vi "Main.vi"() -> ()   [LabVIEW 2020]
uses:
  <vilib>/MakerHub/PS4-Controller/Private/Type Defs/Buttons.ctl
  <vilib>/MakerHub/PS4-Controller/Private/Type Defs/Axis.ctl
  <vilib>/MakerHub/PS4-Controller/Private/Type Defs/Indicators/DPad Enum.ctl
  C:/Users/Public/Documents/Photometrics/PMQI-LabViewSamples/Examples/2018/Dependencies/PVCamNET.dll
  Public/Documents/Photometrics/PMQI-LabViewSamples/Examples/2018/Dependencies/PVCamNET.dll
  <vilib>/SmarAct/SmarActCTL/SA_CTL.lvclass
  <vilib>/MakerHub/PS4-Controller/Private/Type Defs/PS4 Controller Ref.ctl
  <vilib>/Platform/TimedLoop/XDataNode/timing_clust.ctl
  <vilib>/Platform/TimedLoop/XDataNode/nitl_modes.ctl
  <vilib>/Platform/TimedLoop/XDataNode/wakeup.ctl
  <vilib>/platform/TimedLoop/XDataNode/XDataNode.xnode
  <vilib>/Platform/TimedLoop/XDataNode/XDNodeRunTimeDep.lvlib
  <vilib>/MakerHub/PS4-Controller/LMH-PS4.lvlib
panel:
  out "indicator_move_index":dbl
  out "indicator_error":i16
  out "error out 2":errorcluster
  out "indicator_control_sequence":bool=TRUE
  out "indicator_detector_intensity":string="0"
  out "indicator_acquisition_start_time":dbl
  out "indicator_UV_activation_time":dbl
  out "indicator_UV_activation_intensity":dbl
  out "time_out_of_focus":u64 caption="Phidget ID"
  out "indicator_focus_cycle":dbl
  out "indicator_positioner_current_position":i64[](array[numeric])
  out "indicator_focus_searching":bool=TRUE
  out "indicator_focus_userlocked":bool=TRUE
  out "indicator_image_width":u64 caption="Phidget ID"
  out "indicator_LED_power":u64 caption="Phidget ID"
  out "indicator_initial_position_y":u64 caption="Phidget ID"
  out "indicator_initial_position_x":u64 caption="Phidget ID"
  out "indicator_folder_path":string
  out "indicator_saved_positions":i64[][](array[numeric])
  out "indicator_current_position_index":u64 caption="Phidget ID"
  out "indicator_light_source_power":string="2.0"
  out "indicator_red_laser_power":u64 caption="Phidget ID"
  out "indicator_green_laser_power":u64 caption="Phidget ID"
  out "indicator_blue_laser_power":u64 caption="Phidget ID"
  out "indicator_violet_laser_power":u64 caption="Phidget ID"
  out "indicator_current_folder":u64 caption="Phidget ID"
  out "indicator_sequence_distance_y":dbl
  out "indicator_sequence_distance_x":dbl
  out "indicator_sequence_move_y":bool
  out "indicator_sequence_move_x":bool
  out "indicator_current_filter_index":u64 caption="Phidget ID"
  out "indicator_main_positioner_moving_x_y":bool
  in  "control_light_source":string
  out "indicator_devices_reference":T2
  out "indicator_sequence_current_parameters":T3
  out "indicator_sequence_parameters":T4
  out "indicator_camera_buffer_index":u64 caption="Phidget ID"
  in  "control_detector_serial_number":string="69251713"
  out "indicator_joystick_axes":T5
  out "indicator_joystick_buttons":T7
  in  "Stop":bool=TRUE
  out "indicator_main_all_devices_connected":bool
  out "indicator_main_detector_status":bool
  out "indicator_main_filter_status":bool
  out "indicator_main_joystick_status":bool
  out "indicator_main_light sources_status":bool
  out "indicator_main_positioner_status":bool
  out "indicator_main_camera_status":bool
  in  "control_saving_path":path
  out "indicator_message":string="Ready"
  in  "control_frames":string="1000"
  in  "control_sequence":bool
  in  "control_sequence_file_path":path
  in  "control_exposure":string="50"
  out "indicator_focus_status":string="Unfocused"
  out "indicator_x":string
  out "indicator_y":string
  out "indicator_z":string
  out "indicator_light_source":string="Red"
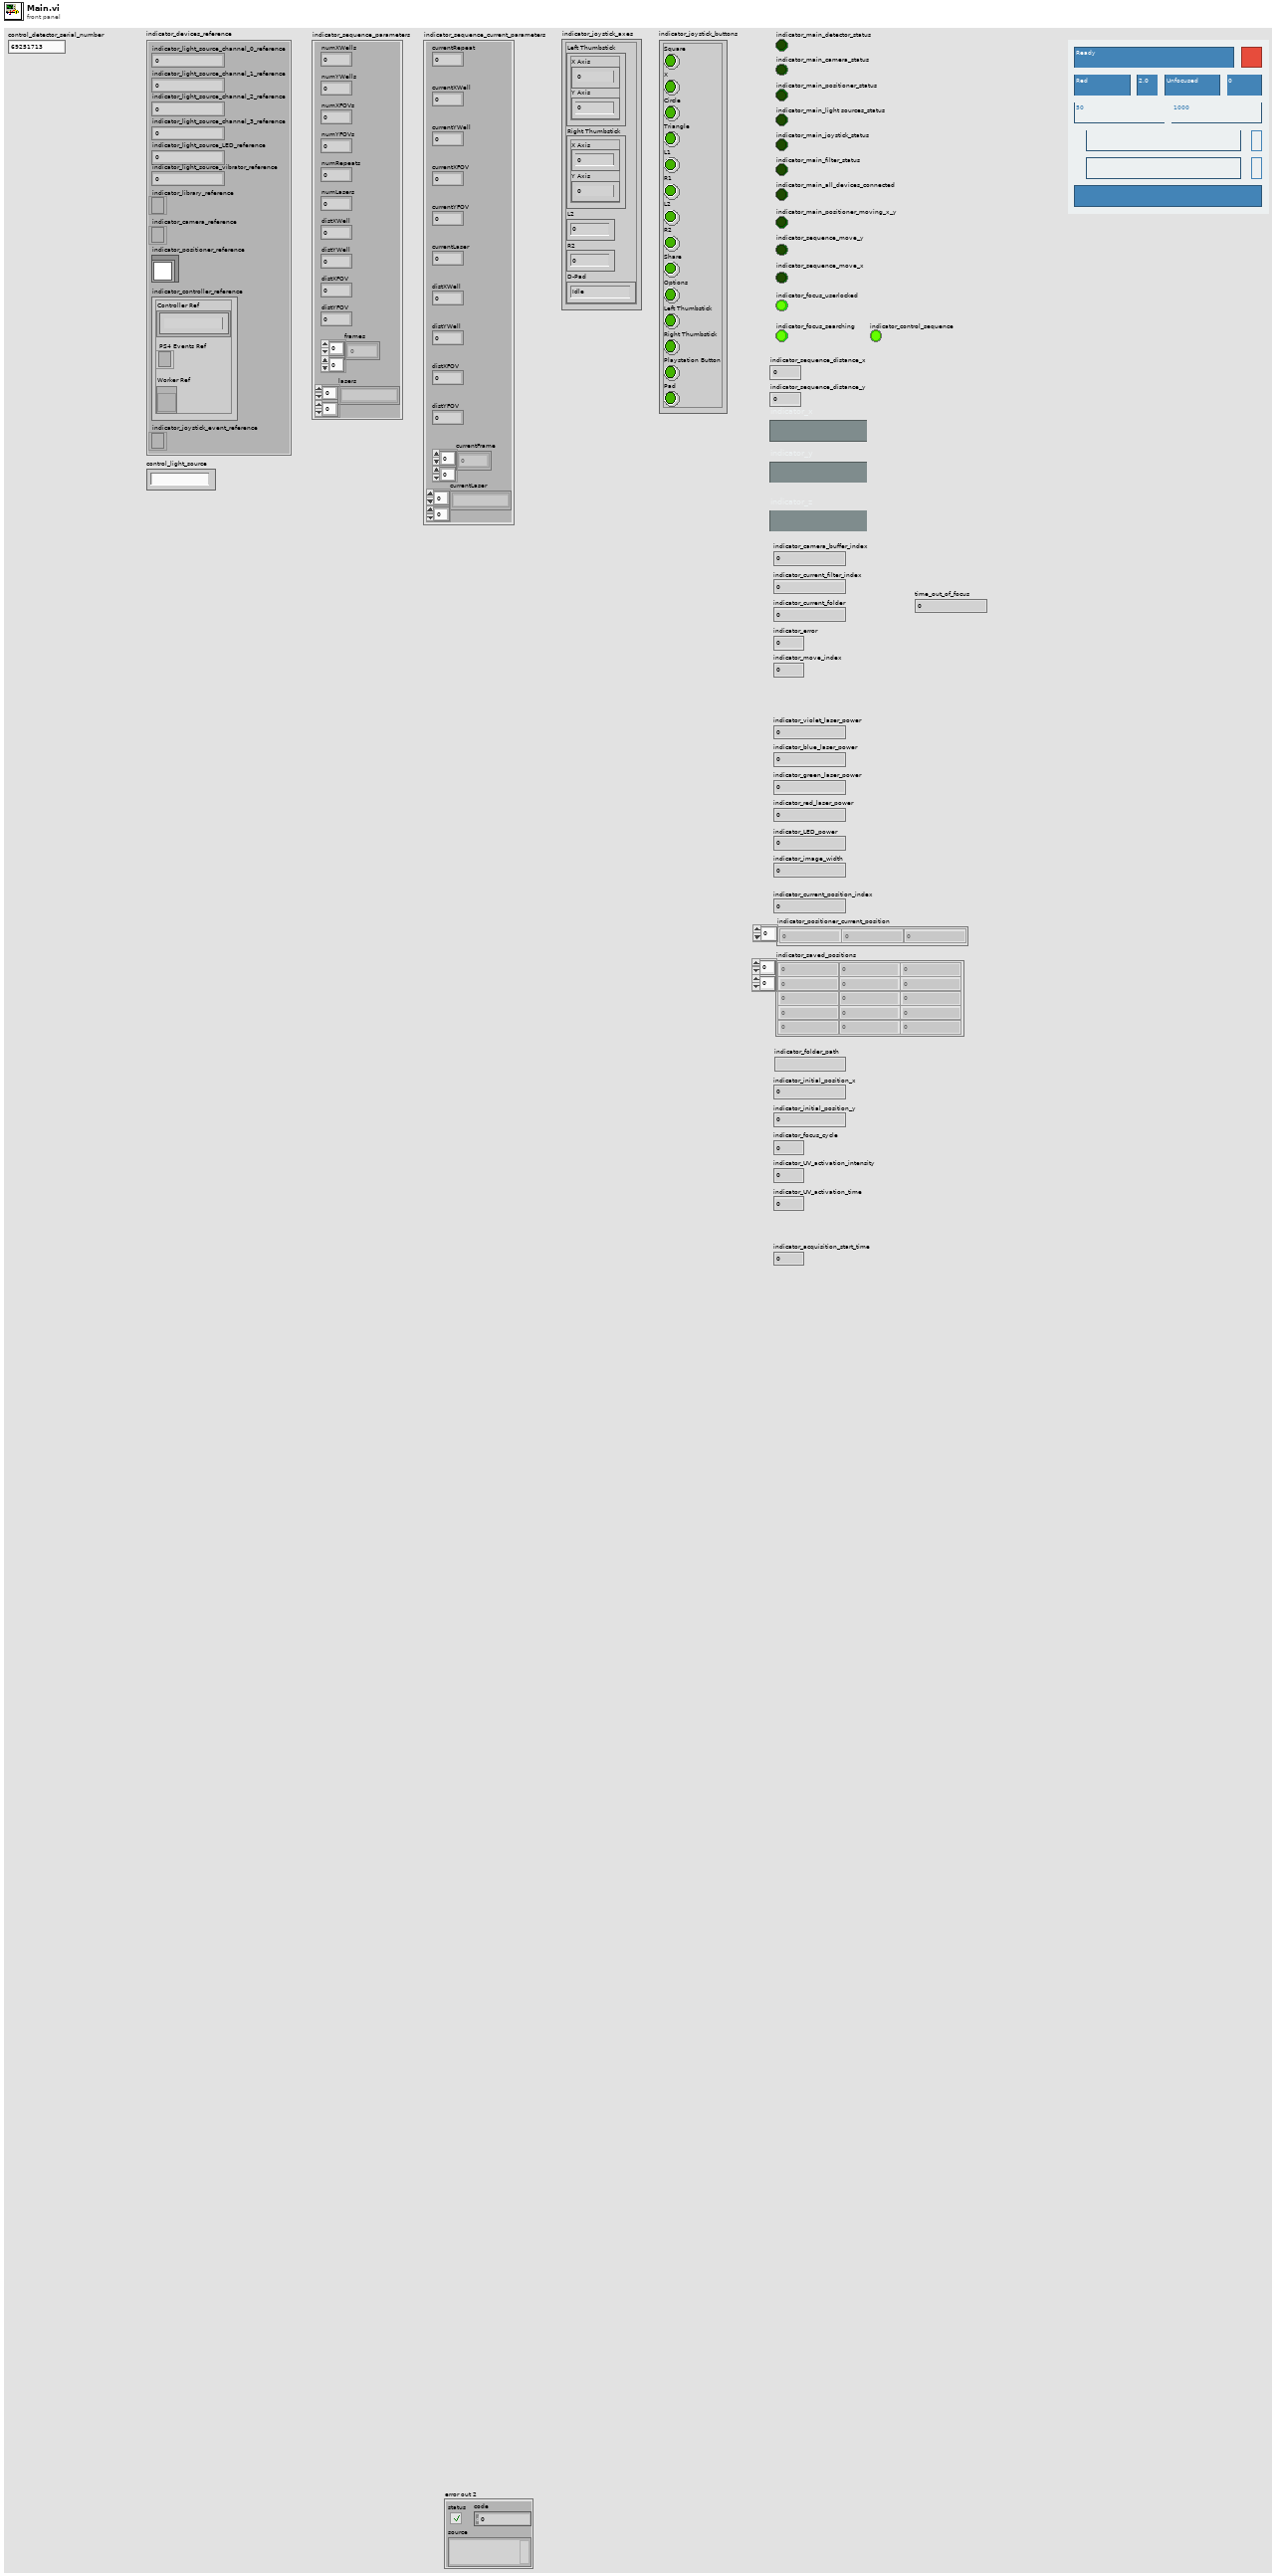
[diagram p1: front panel]
types:
  T1 = typedef "LMH-PS4.lvlib/PS4 Controller Ref.ctl" = cluster{"Controller Ref":refnum<k1>, "PS4 Events Ref":refnum<event-registration>, "Worker Ref":refnum<vi>}
  T2 = cluster{"indicator_light_source_channel_0_reference":u64, "indicator_light_source_channel_1_reference":u64, "indicator_light_source_channel_2_reference":u64, "indicator_light_source_channel_3_reference":u64, "indicator_library_reference":refnum<k24>, "indicator_camera_reference":refnum<k24>, "indicator_positioner_reference":refnum<class "SA_CTL.lvclass">, "indicator_controller_reference":T1, "indicator_joystick_event_reference":refnum<event-registration>, "indicator_light_source_LED_reference":u64, "indicator_light_source_vibrator_reference":u64}
  T3 = cluster{"currentXWell":i32, "currentYWell":i32, "currentXFOV":i32, "currentYFOV":i32, "currentRepeat":i32, "currentLaser":i32, "distXWell":i32, "distYWell":i32, "distXFOV":i32, "distYFOV":i32, "currentFrame":i32[][], "currentLaser":string[][]}
  T4 = cluster{"numXWells":i32, "numYWells":i32, "numXFOVs":i32, "numYFOVs":i32, "numRepeats":i32, "numLasers":i32, "distXWell":i32, "distYWell":i32, "distXFOV":i32, "distYFOV":i32, "frames":i32[][], "lasers":string[][]}
  T5 = typedef "LMH-PS4.lvlib/Axis.ctl" = cluster{"Left Thumbstick":cluster{"X Axis":i32, "Y Axis":i32}, "Right Thumbstick":cluster{"X Axis":i32, "Y Axis":i32}, "L2":i32, "R2":i32, "D-Pad":T6}
  T6 = typedef "LMH-PS4.lvlib/DPad Enum.ctl" = enum16{"Idle", "Up", "Up / Right", "Right", "Down / Right", "Down", "Down / Left", "Left", "Up / Left"}
  T7 = typedef "LMH-PS4.lvlib/Buttons.ctl" = cluster{"Square":bool, "X":bool, "Circle":bool, "Triangle":bool, "L1":bool, "R1":bool, "L2":bool, "R2":bool, "Share":bool, "Options":bool, "Left Thumbstick":bool, "Right Thumbstick":bool, "Playstation Button":bool, "Pad":bool}
  T8 = typedef "XDNodeRunTimeDep.lvlib/timing_clust.ctl" = cluster{"Expected End [f-1]":u64, "Actual End [f-1]":u64, "Finished Late? [f-1]":bool, "Expected End [i-1]":u64, "Actual End [i-1]":u64, "Finished Late? [i-1]":bool, "Expected Start [i]":u64, "Actual Start [i]":u64, "Expected Start [f]":u64, "Actual Start [f]":u64, "Source Name":string, "Structure Name":string, "Period":i64, "Deadline":i64, "Offset":i64, "Start":i64, "Priority":i32, "Timeout":i32, "Mode":T9, "Wakeup Reason":T10, "Error":errorcluster, "Source Type":string, "Secondary Source Type":string, "Global End Time":u64, "Global Start Time":u64, "Frame Duration":u64, "Iteration Duration":u64, "Assigned CPU":i32, "I/O Scan Engine Mode":u32}
  T9 = typedef "XDNodeRunTimeDep.lvlib/nitl_modes.ctl" = enum32{"No Change", "Process missed periods, maintain original phase", "Discard missed periods, maintain original phase", "Process missed periods, ignore original phase", "Discard missed periods, ignore original phase"}
  T10 = typedef "XDNodeRunTimeDep.lvlib/wakeup.ctl" = enum32{"Normal", "Aborted", "Asynchronous wakeup", "Timing source error", "Timed loop error", "Timeout"}
  T11 = cluster{"indicator_light_source_channel_0_reference":u64, "indicator_light_source_channel_1_reference":u64, "indicator_light_source_channel_2_reference":u64, "indicator_light_source_channel_3_reference":u64, "indicator_library_reference":refnum<k24>, "indicator_camera_reference":refnum<k24>, "indicator_positioner_reference":refnum<class "SA_CTL.lvclass">, "indicator_controller_reference":T1, "indicator_joystick_event_reference":refnum<event-registration>, "indicator_light_source_LED_reference":u64, "indicator_light_source_LED_reference 2":u64}
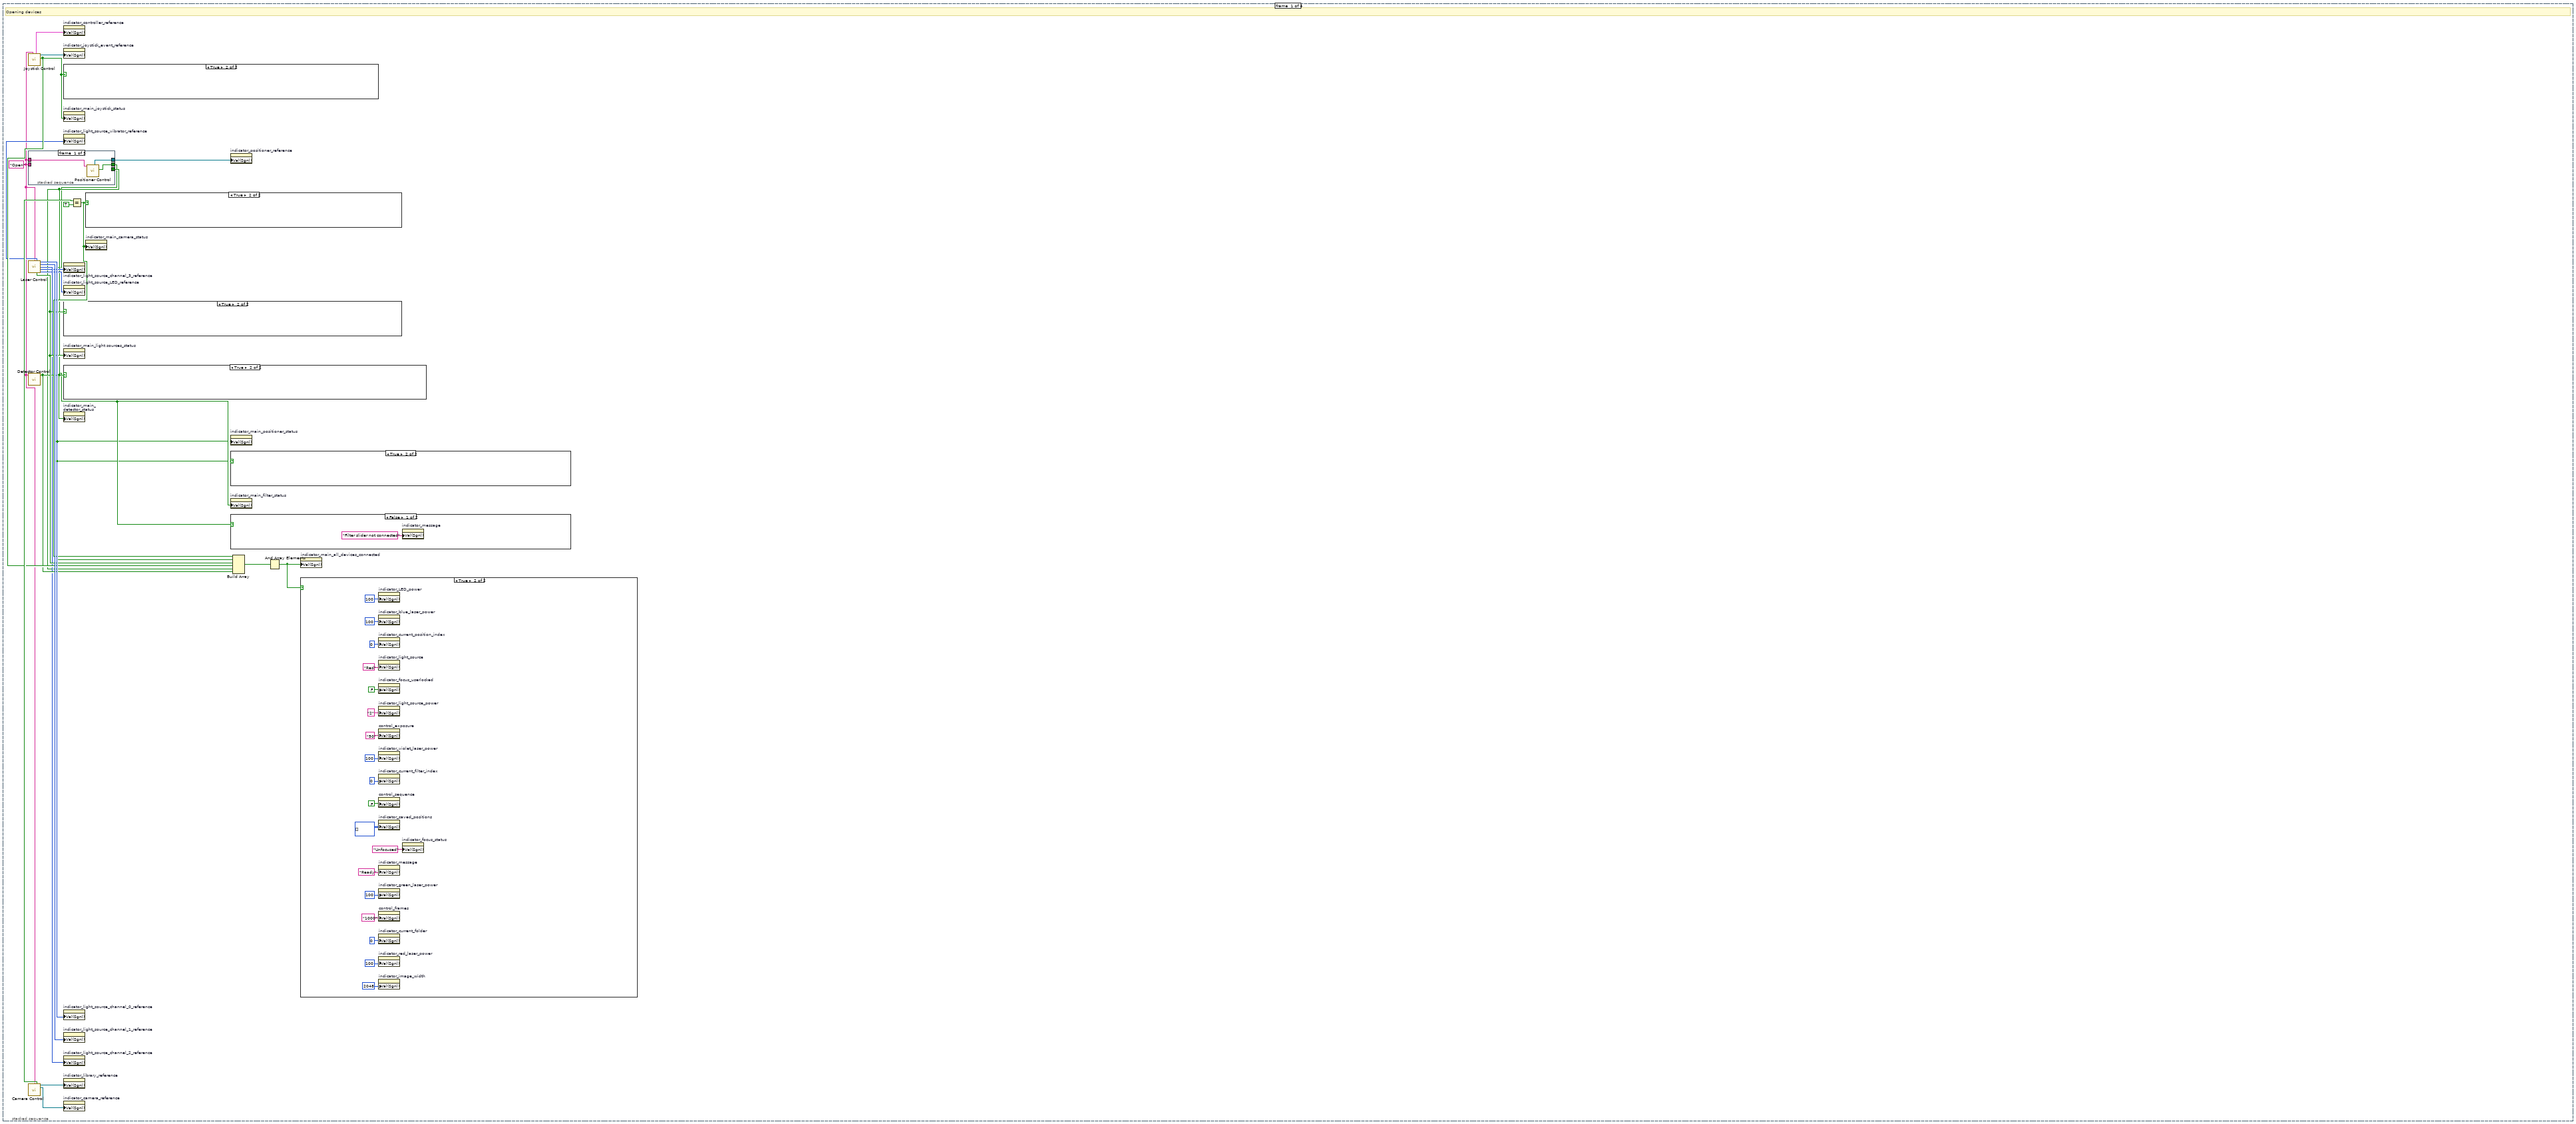
[diagram p2: hidden frame]
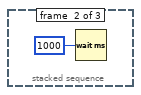
[diagram p3: hidden frame]
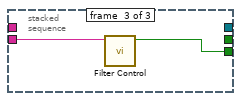
[diagram p4: hidden frame]
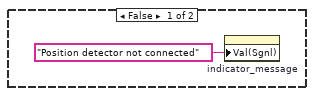
[diagram p6: hidden frame]
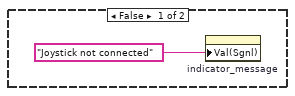
[diagram p8: hidden frame]
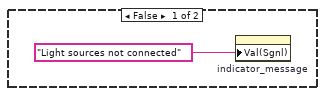
[diagram p9: hidden frame]
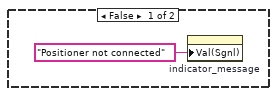
[diagram p10: hidden frame]
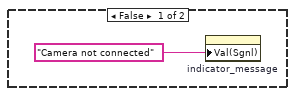
[diagram p11: hidden frame]
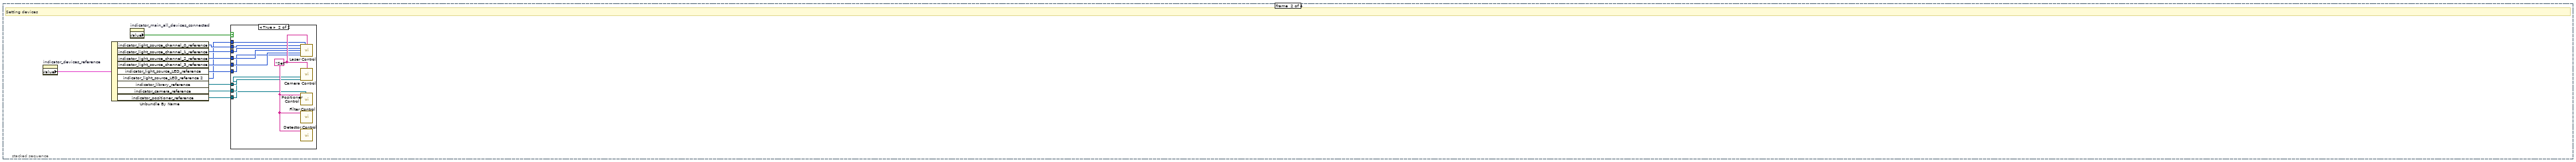
[diagram p12: hidden frame]
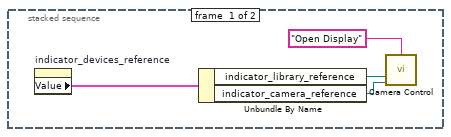
[diagram p15: hidden frame]
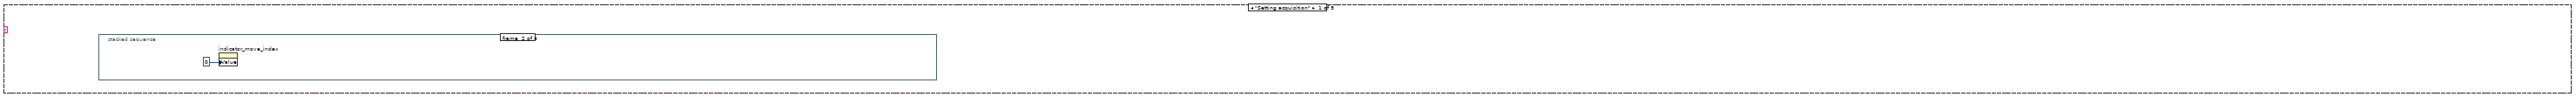
[diagram p16: hidden frame]
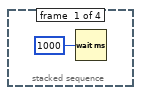
[diagram p17: hidden frame]
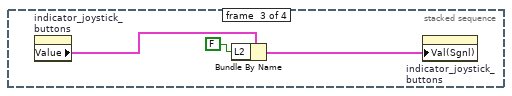
[diagram p18: hidden frame]
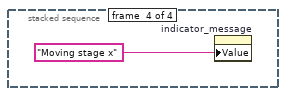
[diagram p19: hidden frame]
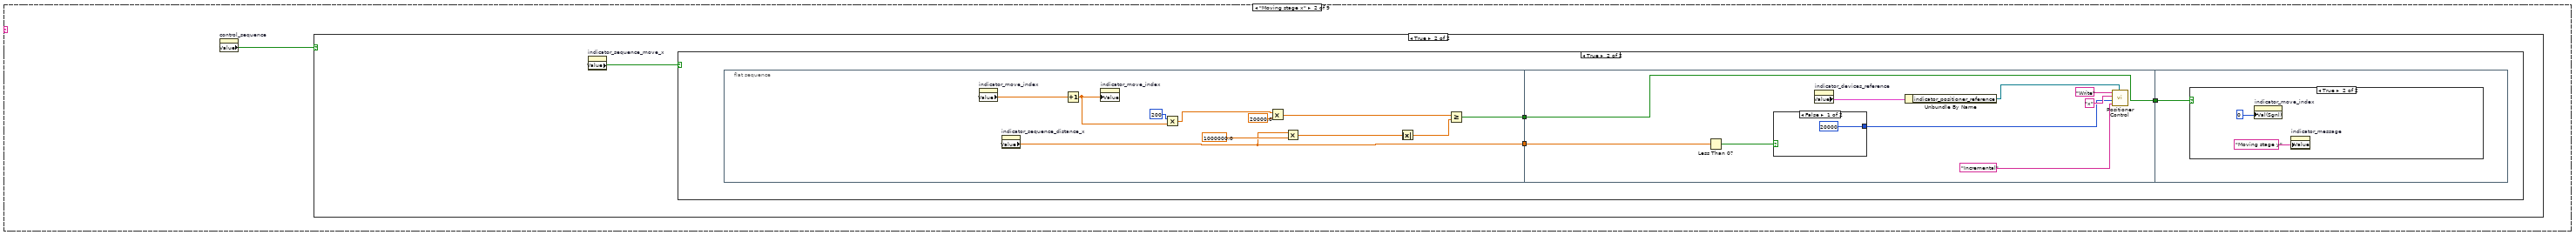
[diagram p20: hidden frame]
diagram:
  n1 = stacked-sequence {
    frame #0 {
      w1 = "Open" ("control_request")
      # "Opening devices"
      n2 = call "Joystick Control.vi"("control_request"=w1) -> ("indicator_joystick_status"=w11:bool, "indicator_joystick_event_reference"=w17:refnum<event-registration>, "indicator_joystick_reference"=w16:T1)  [unwired: 6 in, 2 out]
      n3 = stacked-sequence {
        tunnel: w1 -> [w23 _ _]
        tunnel: [w25 _ _] -> w3
        tunnel: [w24 _ _] -> w2
        tunnel: [_ _ w27] -> w4
        tunnel: w1 -> [_ _ w28]
        frame #0 {
          n4 = call "Positioner Control.vi"("control_request"=w23) -> ("indicator_positioner_status"=w25:bool, "indicator_positioner_reference"=w24:refnum<class "SA_CTL.lvclass">)  [unwired: 5 in, 4 out]
        }
        frame #1 {
          n5 = Wait (ms)(milliseconds to wait=u32 1000) -> ()  [unwired: 1 out]
        }
        frame #2 {
          n6 = call "Filter Control.vi"("control_request"=w28) -> ("indicator_filter_status"=w27:bool)  [unwired: 10 in]
        }
      }
      n7 = call "Laser Control.vi"("control_request"=w1) -> ("indicator_light_source_LED_reference"=w5:u64, "indicator_light_source_channel_0_reference"=w15:u64, "indicator_light_source_channel_1_reference"=w14:u64, "indicator_light_source_channel_2_reference"=w8:u64, "indicator_light_source_channel_3_reference"=w7:u64, "indicator_light_source_status"=w10:bool, "indicator_light_source_vibrator_reference"=w6:u64)  [unwired: 8 in]
      n8 = call "Detector Control.vi"("control_request"=w1) -> ("indicator_detector_status"=w9:bool)  [unwired: 9 in, 1 out]
      n9 = call "Camera Control.vi"("control_request"=w1) -> ("indicator_camera_status"=w22:bool, "indicator_library_reference"=w19:refnum<k24>, "indicator_camera_reference"=w18:refnum<k24>)  [unwired: 10 in, 2 out]
      n10 = property on="indicator_controller_reference" class="Clust (strict)"("Val(Sgnl)"=w16) -> ()  [unwired: 2 in, 2 out]
      n11 = property on="indicator_joystick_event_reference" class="TypRef (strict)"("Val(Sgnl)"=w17) -> ()  [unwired: 2 in, 2 out]
      n12 = case shown="True" w11 {
        frame False {
          n13 = property on="indicator_message" class="Str"("Val(Sgnl)"="Joystick not connected" ("Value (Signaling)")) -> ()  [unwired: 2 in, 2 out]
        }
        frame True {
        }
      }
      n14 = property on="indicator_main_joystick_status" class="Bool (strict)"("Val(Sgnl)"=w11) -> ()  [unwired: 2 in, 2 out]
      n15 = property on="indicator_light_source_vibrator_reference" class="DigNum (strict)"("Val(Sgnl)"=w5) -> ()  [unwired: 2 in, 2 out]
      n16 = property on="indicator_light_source_channel_3_reference" class="DigNum (strict)"("Val(Sgnl)"=w7) -> ()  [unwired: 2 in, 2 out]
      n17 = property on="indicator_light_source_LED_reference" class="DigNum (strict)"("Val(Sgnl)"=w6) -> ()  [unwired: 2 in, 2 out]
      n18 = case shown="True" w10 {
        frame False {
          n19 = property on="indicator_message" class="Str"("Val(Sgnl)"="Light sources not connected" ("Value (Signaling)")) -> ()  [unwired: 2 in, 2 out]
        }
        frame True {
        }
      }
      n20 = property on="indicator_main_light sources_status" class="Bool (strict)"("Val(Sgnl)"=w10) -> ()  [unwired: 2 in, 2 out]
      n21 = case shown="True" w9 {
        frame False {
          n22 = property on="indicator_message" class="Str"("Val(Sgnl)"="Position detector not connected" ("Value (Signaling)")) -> ()  [unwired: 2 in, 2 out]
        }
        frame True {
        }
      }
      n23 = property on="indicator_main_detector_status" class="Bool (strict)"("Val(Sgnl)"=w9) -> ()  [unwired: 2 in, 2 out]
      n24 = property on="indicator_light_source_channel_0_reference" class="DigNum (strict)"("Val(Sgnl)"=w15) -> ()  [unwired: 2 in, 2 out]
      n25 = property on="indicator_light_source_channel_1_reference" class="DigNum (strict)"("Val(Sgnl)"=w14) -> ()  [unwired: 2 in, 2 out]
      n26 = property on="indicator_light_source_channel_2_reference" class="DigNum (strict)"("Val(Sgnl)"=w8) -> ()  [unwired: 2 in, 2 out]
      n27 = property on="indicator_library_reference" class="Ref (strict)"("Val(Sgnl)"=w19) -> ()  [unwired: 2 in, 2 out]
      n28 = property on="indicator_camera_reference" class="Ref (strict)"("Val(Sgnl)"=w18) -> ()  [unwired: 2 in, 2 out]
      n29 = Equal?(x=w22, y=TRUE) -> (x = y?=w13:bool)
      n30 = case shown="True" w13 {
        frame False {
          n31 = property on="indicator_message" class="Str"("Val(Sgnl)"="Camera not connected" ("Value (Signaling)")) -> ()  [unwired: 2 in, 2 out]
        }
        frame True {
        }
      }
      n32 = property on="indicator_main_camera_status" class="Bool (strict)"("Val(Sgnl)"=w13) -> ()  [unwired: 2 in, 2 out]
      n33 = property on="indicator_positioner_reference" class="LVClassControl (strict)"("Val(Sgnl)"=w2) -> ()  [unwired: 2 in, 2 out]
      n34 = property on="indicator_main_positioner_status" class="Bool (strict)"("Val(Sgnl)"=w3) -> ()  [unwired: 2 in, 2 out]
      n35 = case shown="True" w3 {
        frame False {
          n36 = property on="indicator_message" class="Str"("Val(Sgnl)"="Positioner not connected" ("Value (Signaling)")) -> ()  [unwired: 2 in, 2 out]
        }
        frame True {
        }
      }
      n37 = property on="indicator_main_filter_status" class="Bool (strict)"("Val(Sgnl)"=w4) -> ()  [unwired: 2 in, 2 out]
      n38 = case shown="False" w4 {
        frame False {
          n39 = property on="indicator_message" class="Str"("Val(Sgnl)"="Filter slider not connected" ("Value (Signaling)")) -> ()  [unwired: 2 in, 2 out]
        }
        frame True {
        }
      }
      n40 = Build Array(w13, w3, w10, w11, w4, w9) -> (w20:bool[])
      n41 = And Array Elements(Boolean array=w20) -> (logical AND=w12:bool)
      n42 = property on="indicator_main_all_devices_connected" class="Bool (strict)"("Val(Sgnl)"=w12) -> ()  [unwired: 2 in, 2 out]
      n43 = case shown="True" w12 {
        frame False {
        }
        frame True {
          n44 = property on="indicator_LED_power" class="DigNum (strict)"("Val(Sgnl)"=u64 100 ("Value (Signaling)")) -> ()  [unwired: 2 in, 2 out]
          n45 = property on="indicator_blue_laser_power" class="DigNum (strict)"("Val(Sgnl)"=u64 100 ("Value (Signaling)")) -> ()  [unwired: 2 in, 2 out]
          n46 = property on="indicator_current_position_index" class="DigNum (strict)"("Val(Sgnl)"=u64 0 ("Value (Signaling)")) -> ()  [unwired: 2 in, 2 out]
          n47 = property on="indicator_light_source" class="Str"("Val(Sgnl)"="Red" ("Value (Signaling)")) -> ()  [unwired: 2 in, 2 out]
          n48 = property on="indicator_focus_userlocked" class="Bool (strict)"("Val(Sgnl)"=FALSE ("Value (Signaling)")) -> ()  [unwired: 2 in, 2 out]
          n49 = property on="indicator_light_source_power" class="Str"("Val(Sgnl)"="2" ("Value (Signaling)")) -> ()  [unwired: 2 in, 2 out]
          n50 = property on="control_exposure" class="Str"("Val(Sgnl)"="50" ("Value (Signaling)")) -> ()  [unwired: 2 in, 2 out]
          n51 = property on="indicator_violet_laser_power" class="DigNum (strict)"("Val(Sgnl)"=u64 100 ("Value (Signaling)")) -> ()  [unwired: 2 in, 2 out]
          n52 = property on="indicator_current_filter_index" class="DigNum (strict)"("Val(Sgnl)"=u64 0 ("Value (Signaling)")) -> ()  [unwired: 2 in, 2 out]
          n53 = property on="control_sequence" class="Bool (strict)"("Val(Sgnl)"=FALSE ("Value (Signaling)")) -> ()  [unwired: 2 in, 2 out]
          n54 = property on="indicator_saved_positions" class="Arr (strict)"("Val(Sgnl)"=u64[][] [] ("Value (Signaling)")) -> ()  [unwired: 2 in, 2 out]
          n55 = property on="indicator_message" class="Str"("Val(Sgnl)"="Ready" ("Value (Signaling)")) -> ()  [unwired: 2 in, 2 out]
          n56 = property on="indicator_green_laser_power" class="DigNum (strict)"("Val(Sgnl)"=u64 100 ("Value (Signaling)")) -> ()  [unwired: 2 in, 2 out]
          n57 = property on="control_frames" class="Str"("Val(Sgnl)"="1000" ("Value (Signaling)")) -> ()  [unwired: 2 in, 2 out]
          n58 = property on="indicator_current_folder" class="DigNum (strict)"("Val(Sgnl)"=u64 0 ("Value (Signaling)")) -> ()  [unwired: 2 in, 2 out]
          n59 = property on="indicator_red_laser_power" class="DigNum (strict)"("Val(Sgnl)"=u64 100 ("Value (Signaling)")) -> ()  [unwired: 2 in, 2 out]
          n60 = property on="indicator_image_width" class="DigNum (strict)"("Val(Sgnl)"=u64 2048 ("Value (Signaling)")) -> ()  [unwired: 2 in, 2 out]
          n61 = property on="indicator_focus_status" class="Str"("Val(Sgnl)"="Unfocused" ("Value (Signaling)")) -> ()  [unwired: 2 in, 2 out]
        }
      }
    }
    frame #1 {
      # "Setting devices"
      n62 = property on="indicator_devices_reference" class="Clust (strict)"() -> ("Value"=w62:T11)  [unwired: 2 in, 2 out]
      n63 = Unbundle By Name(w62) -> ("indicator_light_source_channel_0_reference"=w61:u64, "indicator_light_source_channel_1_reference"=w60:u64, "indicator_light_source_channel_2_reference"=w59:u64, "indicator_light_source_channel_3_reference"=w58:u64, "indicator_light_source_LED_reference"=w54:u64, "indicator_light_source_LED_reference 2"=w53:u64, "indicator_library_reference"=w56:refnum<k24>, "indicator_camera_reference"=w55:refnum<k24>, "indicator_positioner_reference"=w57:refnum<class "SA_CTL.lvclass">)
      n64 = property on="indicator_main_all_devices_connected" class="Bool (strict)"() -> ("Value"=w63:bool)  [unwired: 2 in, 2 out]
      n65 = case shown="True" w63 {
        tunnel: w56 -> [_ w72]
        tunnel: w55 -> [_ w71]
        tunnel: w57 -> [_ w70]
        tunnel: w61 -> [_ w69]
        tunnel: w60 -> [_ w68]
        tunnel: w59 -> [_ w67]
        tunnel: w58 -> [_ w66]
        tunnel: w54 -> [_ w65]
        tunnel: w53 -> [_ w64]
        frame False {
        }
        frame True {
          w73 = "Set" ("control_request")
          n66 = call "Laser Control.vi"("control_laser_source_channel_0_reference"=w69, "control_laser_source_LED_reference"=w64, "control_request"=w73, "control_laser_source_channel_1_reference"=w68, "control_laser_source_channel_2_reference"=w67, "control_laser_source_channel_3_reference"=w66, "control_laser_source_vibrator_reference"=w65) -> ()  [unwired: 2 in, 7 out]
          n67 = call "Camera Control.vi"("control_request"=w73, "control_library_reference"=w72, "control_camera_reference"=w71) -> ()  [unwired: 8 in, 5 out]
          n68 = call "Positioner Control.vi"("control_positioner_reference"=w70, "control_request"=w73) -> ()  [unwired: 4 in, 6 out]
          n69 = call "Filter Control.vi"("control_request"=w73) -> ()  [unwired: 10 in, 1 out]
          n70 = call "Detector Control.vi"("control_request"=w73) -> ()  [unwired: 9 in, 2 out]
        }
      }
    }
    frame #2 {
      # "Main loop"
      n71 = property on="indicator_main_all_devices_connected" class="Bool (strict)"() -> ("Value"=w74:bool)  [unwired: 2 in, 2 out]
      n72 = case shown="True" w74 {
        frame False {
        }
        frame True {
          n73 = stacked-sequence {
            frame #0 {
              n74 = property on="indicator_devices_reference" class="Clust (strict)"() -> ("Value"=w78:T11)  [unwired: 2 in, 2 out]
              n75 = Unbundle By Name(w78) -> ("indicator_library_reference"=w77:refnum<k24>, "indicator_camera_reference"=w76:refnum<k24>)
              n76 = call "Camera Control.vi"("control_request"="Open Display", "control_library_reference"=w77, "control_camera_reference"=w76) -> ()  [unwired: 8 in, 5 out]
            }
            frame #1 {
              n77 = node-c288(i64 10 ("Period")) -> (w81:T8)  [unwired: 3 in]
              n78 = timed-loop {
                timing: w81 -> [_]
                timing-out: [_] -> w80
                i -> [w85]
                stop <- "Stop" continue-if-true
                n79 = node-c288() -> ()  [unwired: 1 in, 1 out]
                n80 = property on="D-Pad" class="Enum (strict)"() -> ("Value"=w106:T6)  [unwired: 2 in, 2 out]
                n81 = Quotient & Remainder(x=w85, y=20) -> (x-y*floor(x/y)=w83:i32)  [unwired: 1 out]
                n82 = Equal To 0?(x=w83) -> ()  [unwired: 1 out]
                n83 = case shown="\"Down\"" w106 {
                  frame "Idle", Default {
                  }
                  frame "Up" {
                    n84 = stacked-sequence {
                      seq-local: [w469 _ _ _ _ _] -> [_ w476 _ _ _ _]
                      seq-local: [_ w476 _ _ _ _] -> [_ _ w480 _ _ _]
                      seq-local: [_ w475 _ _ _ _] -> [_ _ w477 _ _ _]
                      seq-local: [_ _ w477 _ _ _] -> [_ _ _ w483 _ _]
                      seq-local: [_ _ _ w483 _ _] -> [_ _ _ _ _ w486]
                      frame #0 {
                        n85 = property on="indicator_saved_positions" class="Arr (strict)"() -> ("Value"=w472:i64[][])  [unwired: 2 in, 2 out]
                        n86 = Array Size(array=w472) -> (size(s)=w474:i32[])
                        n87 = property on="indicator_positioner_current_position" class="Arr (strict)"() -> ("Value"=w471:i64[])  [unwired: 2 in, 2 out]
                        n88 = Index Array(array=w474, index=0) -> (element=w468:i32)
                        n89 = property on="indicator_current_position_index" class="DigNum (strict)"("Val(Sgnl)"=w468) -> ()  [unwired: 2 in, 2 out]
                        n90 = Insert Into Array(array=w472, index (row)=w468, new element=w471) -> (w470:i64[][])  [unwired: 1 in]
                        n91 = property on="indicator_saved_positions" class="Arr (strict)"("Val(Sgnl)"=w470) -> ()  [unwired: 2 in, 2 out]
                        n92 = Increment(x=w468) -> (x+1=w469:i32)
                      }
                      frame #1 {
                        n93 = property on="indicator_message" class="Str"() -> ("Value"=w475:string)  [unwired: 2 in, 2 out]
                      }
                      frame #2 {
                        n94 = Number To Decimal String(number=w480) -> (decimal integer string=w481:string)  [unwired: 1 in]
                        n95 = Concatenate Strings("Position number " ("string"), w481, " added" ("string")) -> (w478:string)
                        n96 = property on="indicator_message" class="Str"("Val(Sgnl)"=w478) -> ()  [unwired: 2 in, 2 out]
                      }
                      frame #3 {
                        n97 = Wait (ms)(milliseconds to wait=u32 1000) -> ()  [unwired: 1 out]
                      }
                      frame #4 {
                        n98 = property on="D-Pad" class="Enum (strict)"("Val(Sgnl)"=DPad_Enum."Idle" ("Value (Signaling)")) -> ()  [unwired: 2 in, 2 out]
                      }
                      frame #5 {
                        n99 = property on="indicator_message" class="Str"("Val(Sgnl)"=w486) -> ()  [unwired: 2 in, 2 out]
                      }
                    }
                  }
                  frame "Down" {
                    n100 = stacked-sequence {
                      seq-local: [w488 _ _ _ _ _] -> [_ w497 _ _ _ _]
                      seq-local: [w487 _ _ _ _ _] -> [_ w496 _ _ _ _]
                      seq-local: [_ w498 _ _ _ _] -> [_ _ w501 _ _ _]
                      seq-local: [_ w497 _ _ _ _] -> [_ _ w500 _ _ _]
                      seq-local: [_ w496 _ _ _ _] -> [_ _ w499 _ _ _]
                      seq-local: [_ _ w501 _ _ _] -> [_ _ _ w509 _ _]
                      seq-local: [_ _ _ w509 _ _] -> [_ _ _ _ _ w512]
                      frame #0 {
                        n101 = property on="indicator_saved_positions" class="Arr (strict)"() -> ("Value"=w489:i64[][])  [unwired: 2 in, 2 out]
                        n102 = Array Size(array=w489) -> (size(s)=w491:i32[])
                        n103 = Index Array(array=w491, index=0) -> (element=w488:i32)
                        n104 = Greater Than 0?(x=w488) -> (x > 0?=w487:bool)
                        n105 = case shown="True" w487 {
                          tunnel: w489 -> [_ w495]
                          tunnel: w488 -> [_ w493]
                          frame False {
                          }
                          frame True {
                            n106 = Decrement(x=w493) -> (x-1=w492:i32)
                            n107 = property on="indicator_current_position_index" class="DigNum (strict)"("Val(Sgnl)"=w492) -> ()  [unwired: 2 in, 2 out]
                            n108 = Delete From Array(array=w495, index (row)=w492) -> (array with subset deleted=w494:i64[][])  [unwired: 2 in, 1 out]
                            n109 = property on="indicator_saved_positions" class="Arr (strict)"("Val(Sgnl)"=w494) -> ()  [unwired: 2 in, 2 out]
                          }
                        }
                      }
                      frame #1 {
                        n110 = property on="indicator_message" class="Str"() -> ("Value"=w498:string)  [unwired: 2 in, 2 out]
                      }
                      frame #2 {
                        n111 = case shown="True" w499 {
                          tunnel: ["No positions to remove" w505] -> w502
                          tunnel: w500 -> [_ w504]
                          frame False {
                          }
                          frame True {
                            n112 = Number To Decimal String(number=w504) -> (decimal integer string=w507:string)  [unwired: 1 in]
                            n113 = Concatenate Strings("Position number " ("string"), w507, " removed" ("string")) -> (w505:string)
                          }
                        }
                        n114 = property on="indicator_message" class="Str"("Val(Sgnl)"=w502) -> ()  [unwired: 2 in, 2 out]
                      }
                      frame #3 {
                        n115 = Wait (ms)(milliseconds to wait=u32 1000) -> ()  [unwired: 1 out]
                      }
                      frame #4 {
                        n116 = property on="D-Pad" class="Enum (strict)"("Val(Sgnl)"=DPad_Enum."Idle" ("Value (Signaling)")) -> ()  [unwired: 2 in, 2 out]
                      }
                      frame #5 {
                        n117 = property on="indicator_message" class="Str"("Val(Sgnl)"=w512) -> ()  [unwired: 2 in, 2 out]
                      }
                    }
                  }
                  frame "Left" {
                    n118 = property on="indicator_message" class="Str"() -> ("Value"=w515:string)  [unwired: 2 in, 2 out]
                    n119 = Equal?(x=w515, y="Live") -> (x = y?=w517:bool)
                    n120 = Equal?(x=w515, y="Ready") -> (x = y?=w516:bool)
                    n121 = Or(x=w517, y=w516) -> (x .or. y?=w513:bool)
                    n122 = case shown="True" w513 {
                      frame False {
                      }
                      frame True {
                        n123 = stacked-sequence {
                          seq-local: [w530 _ _ _ _ _] -> [_ w566 _ _ _ _]
                          seq-local: [w519 _ _ _ _ _] -> [_ w565 _ _ _ _]
                          seq-local: [_ w567 _ _ _ _] -> [_ _ w568 _ _ _]
                          seq-local: [_ w566 _ _ _ _] -> [_ _ w570 _ _ _]
                          seq-local: [_ w565 _ _ _ _] -> [_ _ w569 _ _ _]
                          seq-local: [_ _ w568 _ _ _] -> [_ _ _ w577 _ _]
                          seq-local: [_ _ w569 _ _ _] -> [_ _ _ w578 _ _]
                          seq-local: [_ _ _ w577 _ _] -> [_ _ _ _ w589 _]
                          seq-local: [_ _ _ _ w589 _] -> [_ _ _ _ _ w590]
                          frame #0 {
                            n124 = property on="indicator_saved_positions" class="Arr (strict)"() -> ("Value"=w527:i64[][])  [unwired: 2 in, 2 out]
                            n125 = Array Size(array=w527) -> (size(s)=w529:i32[])
                            n126 = property on="indicator_current_position_index" class="DigNum (strict)"() -> ("Value"=w531:u64)  [unwired: 2 in, 2 out]
                            n127 = Index Array(array=w529, index=0) -> (element=w526:i32)
                            n128 = Decrement(x=w526) -> (x-1=w525:i32)
                            n129 = Decrement(x=w531) -> (x-1=w520:u64)
                            n130 = To Quad Integer(1:w525) -> (0:w524:i64)
                            n131 = To Quad Integer(1:w520) -> (0:w521:i64)
                            n132 = To Quad Integer(1:u64 0 ("lower limit")) -> (0:w522:i64)
                            n133 = In Range and Coerce(upper limit=w524, x=w521, lower limit=w522) -> (coerced(x)=w530:i64, In Range?=w519:bool)
                            n134 = case shown="True" w519 {
                              tunnel: w527 -> [_ w557]
                              tunnel: w530 -> [_ w556]
                              frame False {
                              }
                              frame True {
                                n135 = Index Array(array=w557, index (row)=w556, index (col)=2 ("disabled index (col)")) -> (element=w546:i64)
                                n136 = Index Array(array=w557, index (row)=w556, index (col)=1 ("disabled index (col)")) -> (element=w548:i64)
                                n137 = Index Array(array=w557, index (row)=w556, index (col)=0 ("disabled index (col)")) -> (element=w550:i64)
                                n138 = property on="indicator_positioner_current_position" class="Arr (strict)"() -> ("Value"=w552:i64[])  [unwired: 2 in, 2 out]
                                n139 = property on="indicator_focus_status" class="Str"() -> ("Value"=w536:string)  [unwired: 2 in, 2 out]
                                n140 = Index Array(array=w552, index=2) -> (element=w545:i64)
                                n141 = Index Array(array=w552, index=1) -> (element=w547:i64)
                                n142 = Index Array(array=w552, index=0) -> (element=w549:i64)
                                n143 = property on="indicator_positioner_reference" class="LVClassControl (strict)"() -> ("Value"=w533:refnum<class "SA_CTL.lvclass">)  [unwired: 2 in, 2 out]
                                n144 = Equal?(x=w536, y="Locked") -> (x = y?=w534:bool)
                                n145 = Subtract(x=w546, y=w545) -> (x-y=w532:i64)
                                n146 = Subtract(x=w548, y=w547) -> (x-y=w537:i64)
                                n147 = Subtract(x=w550, y=w549) -> (x-y=w541:i64)
                                n148 = case shown="False" w534 {
                                tunnel: w533 -> [w561 _]
                                tunnel: w532 -> [w560 _]
                                frame False {
                                n149 = call "Positioner Control.vi"("control_move_length"=w560, "control_positioner_reference"=w561, "mode"="Set", "control_move_direction"="z", "control_request"="Write") -> ()  [unwired: 1 in, 6 out]
                                }
                                frame True {
                                }
                                }
                                n150 = call "Positioner Control.vi"("control_move_length"=w537, "control_positioner_reference"=w533, "mode"="Set", "control_move_direction"="y", "control_request"="Write") -> ()  [unwired: 1 in, 6 out]
                                n151 = call "Positioner Control.vi"("control_move_length"=w541, "control_positioner_reference"=w533, "mode"="Set", "control_move_direction"="x", "control_request"="Write") -> ()  [unwired: 1 in, 6 out]
                              }
                            }
                            n152 = property on="indicator_current_position_index" class="DigNum (strict)"("Val(Sgnl)"=w530) -> ()  [unwired: 2 in, 2 out]
                          }
                          frame #1 {
                            n153 = property on="indicator_message" class="Str"() -> ("Value"=w567:string)  [unwired: 2 in, 2 out]
                          }
                          frame #2 {
                            n154 = case shown="True" w569 {
                              tunnel: ["First position reached" w574] -> w571
                              tunnel: w570 -> [_ w573]
                              frame False {
                              }
                              frame True {
                                n155 = Number To Decimal String(number=w573) -> (decimal integer string=w575:string)  [unwired: 1 in]
                                n156 = Concatenate Strings("Moving to position number " ("string"), w575) -> (w574:string)
                              }
                            }
                            n157 = property on="indicator_message" class="Str"("Val(Sgnl)"=w571) -> ()  [unwired: 2 in, 2 out]
                          }
                          frame #3 {
                            n158 = case shown="False" w578 {
                              frame False {
                                n159 = Wait (ms)(milliseconds to wait=u32 1000) -> ()  [unwired: 1 out]
                              }
                              frame True {
                                n160 = stacked-sequence {
                                frame #0 {
                                n161 = while {
                                stop <- w580 continue-if-true
                                n162 = property on="indicator_positioner_reference" class="LVClassControl (strict)"() -> ("Value"=w585:refnum<class "SA_CTL.lvclass">)  [unwired: 2 in, 2 out]
                                n163 = call "Positioner Control.vi"("control_positioner_reference"=w585, "control_request"="Is Moving") -> ("indicator_positioner_ismoving_y"=w583:bool, "indicator_positioner_ismoving_x"=w584:bool, "indicator_positioner_ismoving_z"=w582:bool)  [unwired: 4 in, 3 out]
                                n164 = Build Array(w584, w583, w582) -> (w581:bool[])
                                n165 = Or Array Elements(Boolean array=w581) -> (logical OR=w580:bool)
                                }
                                }
                                frame #1 {
                                n166 = Wait (ms)(milliseconds to wait=u32 1000) -> ()  [unwired: 1 out]
                                }
                                }
                              }
                            }
                          }
                          frame #4 {
                            n167 = property on="D-Pad" class="Enum (strict)"("Val(Sgnl)"=DPad_Enum."Idle" ("Value (Signaling)")) -> ()  [unwired: 2 in, 2 out]
                          }
                          frame #5 {
                            n168 = property on="indicator_message" class="Str"("Val(Sgnl)"=w590) -> ()  [unwired: 2 in, 2 out]
                          }
                        }
                      }
                    }
                  }
                  frame "Right" {
                    # "Registering / Deleting Positioners Position For Use in Acquiring"
                    n169 = stacked-sequence {
                      seq-local: [w602 _ _ _ _ _] -> [_ w638 _ _ _ _]
                      seq-local: [w591 _ _ _ _ _] -> [_ w637 _ _ _ _]
                      seq-local: [_ w639 _ _ _ _] -> [_ _ w640 _ _ _]
                      seq-local: [_ w638 _ _ _ _] -> [_ _ w642 _ _ _]
                      seq-local: [_ w637 _ _ _ _] -> [_ _ w641 _ _ _]
                      seq-local: [_ _ w640 _ _ _] -> [_ _ _ w649 _ _]
                      seq-local: [_ _ w641 _ _ _] -> [_ _ _ w650 _ _]
                      seq-local: [_ _ _ w649 _ _] -> [_ _ _ _ w661 _]
                      seq-local: [_ _ _ _ w661 _] -> [_ _ _ _ _ w662]
                      frame #0 {
                        n170 = property on="indicator_saved_positions" class="Arr (strict)"() -> ("Value"=w599:i64[][])  [unwired: 2 in, 2 out]
                        n171 = Array Size(array=w599) -> (size(s)=w601:i32[])
                        n172 = property on="indicator_current_position_index" class="DigNum (strict)"() -> ("Value"=w603:u64)  [unwired: 2 in, 2 out]
                        n173 = Index Array(array=w601, index=0) -> (element=w598:i32)
                        n174 = Decrement(x=w598) -> (x-1=w597:i32)
                        n175 = Increment(x=w603) -> (x+1=w592:u64)
                        n176 = To Quad Integer(1:w597) -> (0:w596:i64)
                        n177 = To Quad Integer(1:w592) -> (0:w593:i64)
                        n178 = To Quad Integer(1:u64 0 ("lower limit")) -> (0:w594:i64)
                        n179 = In Range and Coerce(upper limit=w596, x=w593, lower limit=w594) -> (coerced(x)=w602:i64, In Range?=w591:bool)
                        n180 = case shown="True" w591 {
                          tunnel: w599 -> [_ w629]
                          tunnel: w602 -> [_ w628]
                          frame False {
                          }
                          frame True {
                            n181 = Index Array(array=w629, index (row)=w628, index (col)=2 ("disabled index (col)")) -> (element=w618:i64)
                            n182 = Index Array(array=w629, index (row)=w628, index (col)=1 ("disabled index (col)")) -> (element=w620:i64)
                            n183 = Index Array(array=w629, index (row)=w628, index (col)=0 ("disabled index (col)")) -> (element=w622:i64)
                            n184 = property on="indicator_positioner_current_position" class="Arr (strict)"() -> ("Value"=w624:i64[])  [unwired: 2 in, 2 out]
                            n185 = property on="indicator_focus_status" class="Str"() -> ("Value"=w608:string)  [unwired: 2 in, 2 out]
                            n186 = Index Array(array=w624, index=2) -> (element=w617:i64)
                            n187 = Index Array(array=w624, index=1) -> (element=w619:i64)
                            n188 = Index Array(array=w624, index=0) -> (element=w621:i64)
                            n189 = property on="indicator_positioner_reference" class="LVClassControl (strict)"() -> ("Value"=w605:refnum<class "SA_CTL.lvclass">)  [unwired: 2 in, 2 out]
                            n190 = Equal?(x=w608, y="Locked") -> (x = y?=w606:bool)
                            n191 = Subtract(x=w618, y=w617) -> (x-y=w604:i64)
                            n192 = Subtract(x=w620, y=w619) -> (x-y=w609:i64)
                            n193 = Subtract(x=w622, y=w621) -> (x-y=w613:i64)
                            n194 = case shown="False" w606 {
                              tunnel: w605 -> [w633 _]
                              tunnel: w604 -> [w632 _]
                              frame False {
                                n195 = call "Positioner Control.vi"("control_move_length"=w632, "control_positioner_reference"=w633, "mode"="Set", "control_move_direction"="z", "control_request"="Write") -> ()  [unwired: 1 in, 6 out]
                              }
                              frame True {
                              }
                            }
                            n196 = call "Positioner Control.vi"("control_move_length"=w609, "control_positioner_reference"=w605, "mode"="Set", "control_move_direction"="y", "control_request"="Write") -> ()  [unwired: 1 in, 6 out]
                            n197 = call "Positioner Control.vi"("control_move_length"=w613, "control_positioner_reference"=w605, "mode"="Set", "control_move_direction"="x", "control_request"="Write") -> ()  [unwired: 1 in, 6 out]
                          }
                        }
                        n198 = property on="indicator_current_position_index" class="DigNum (strict)"("Val(Sgnl)"=w602) -> ()  [unwired: 2 in, 2 out]
                      }
                      frame #1 {
                        n199 = property on="indicator_message" class="Str"() -> ("Value"=w639:string)  [unwired: 2 in, 2 out]
                      }
                      frame #2 {
                        n200 = case shown="False" w641 {
                          tunnel: ["Last position reached" w646] -> w643
                          tunnel: w642 -> [_ w645]
                          frame False {
                          }
                          frame True {
                            n201 = Number To Decimal String(number=w645) -> (decimal integer string=w647:string)  [unwired: 1 in]
                            n202 = Concatenate Strings("Moving to position number " ("string"), w647) -> (w646:string)
                          }
                        }
                        n203 = property on="indicator_message" class="Str"("Val(Sgnl)"=w643) -> ()  [unwired: 2 in, 2 out]
                      }
                      frame #3 {
                        n204 = case shown="True" w650 {
                          frame False {
                            n205 = Wait (ms)(milliseconds to wait=u32 2000) -> ()  [unwired: 1 out]
                          }
                          frame True {
                            n206 = flat-sequence {
                              frame #0 {
                                n207 = while {
                                stop <- w652 continue-if-true
                                n208 = property on="indicator_positioner_reference" class="LVClassControl (strict)"() -> ("Value"=w657:refnum<class "SA_CTL.lvclass">)  [unwired: 2 in, 2 out]
                                n209 = call "Positioner Control.vi"("control_positioner_reference"=w657, "control_request"="Is Moving") -> ("indicator_positioner_ismoving_y"=w655:bool, "indicator_positioner_ismoving_x"=w656:bool, "indicator_positioner_ismoving_z"=w654:bool)  [unwired: 4 in, 3 out]
                                n210 = Build Array(w656, w655, w654) -> (w653:bool[])
                                n211 = Or Array Elements(Boolean array=w653) -> (logical OR=w652:bool)
                                }
                              }
                              frame #1 {
                                n212 = Wait (ms)(milliseconds to wait=u32 1000) -> ()  [unwired: 1 out]
                              }
                            }
                          }
                        }
                      }
                      frame #4 {
                        n213 = property on="D-Pad" class="Enum (strict)"("Val(Sgnl)"=DPad_Enum."Idle" ("Value (Signaling)")) -> ()  [unwired: 2 in, 2 out]
                      }
                      frame #5 {
                        n214 = property on="indicator_message" class="Str"("Val(Sgnl)"=w662) -> ()  [unwired: 2 in, 2 out]
                      }
                    }
                  }
                }
                n215 = property on="indicator_joystick_axes" class="Clust (strict)"() -> ("Value"=w139:T5)  [unwired: 2 in, 2 out]
                n216 = property on="control_saving_path" class="Path"() -> ("Value"=w143:path)  [unwired: 2 in, 2 out]
                n217 = property on="indicator_message" class="Str"() -> ("Value"=w82:string)  [unwired: 2 in, 2 out]
                n218 = call "Detector Control.vi"("control_request"="Read") -> ("indicator_detector_reading"=w125:cluster{"x":i16, "y":i16, "sum":u16})  [unwired: 9 in, 1 out]
                n219 = property on="indicator_positioner_reference" class="LVClassControl (strict)"() -> ("Value"=w112:refnum<class "SA_CTL.lvclass">)  [unwired: 2 in, 2 out]
                n220 = Unbundle By Name(w139) -> ("Right Thumbstick.X Axis"=w127:i32, "Right Thumbstick.Y Axis"=w130:i32, "Left Thumbstick.Y Axis"=w131:i32, "Left Thumbstick.X Axis"=w134:i32)
                n221 = case shown="\"Stabilizing\"" w82 {
                  frame "Setting acquisition" {
                    n222 = stacked-sequence {
                      frame #0 {
                        n223 = Wait (ms)(milliseconds to wait=u32 1000) -> ()  [unwired: 1 out]
                      }
                      frame #1 {
                        n224 = property on="indicator_move_index" class="DigNum (strict)"("Value"=i16 0 ("indicator_move_index")) -> ()  [unwired: 2 in, 2 out]
                      }
                      frame #2 {
                        n225 = property on="indicator_joystick_buttons" class="Clust (strict)"() -> ("Value"=w189:T7)  [unwired: 2 in, 2 out]
                        n226 = Bundle By Name(cluster=w189, "L2"=FALSE ("R1")) -> (w190:T7)
                        n227 = property on="indicator_joystick_buttons" class="Clust (strict)"("Val(Sgnl)"=w190) -> ()  [unwired: 2 in, 2 out]
                      }
                      frame #3 {
                        n228 = property on="indicator_message" class="Str"("Value"="Moving stage x" ("indicator_message")) -> ()  [unwired: 2 in, 2 out]
                      }
                    }
                  }
                  frame "Moving stage x" {
                    n229 = property on="control_sequence" class="Bool (strict)"() -> ("Value"=w192:bool)  [unwired: 2 in, 2 out]
                    n230 = case shown="True" w192 {
                      frame False {
                        n231 = property on="indicator_message" class="Str"("Value"="Starting acquisition" ("indicator_message")) -> ()  [unwired: 2 in, 2 out]
                      }
                      frame True {
                        n232 = property on="indicator_sequence_move_x" class="Bool (strict)"() -> ("Value"=w194:bool)  [unwired: 2 in, 2 out]
                        n233 = case shown="True" w194 {
                          frame False {
                            n234 = property on="indicator_message" class="Str"("Value"="Moving stage y" ("indicator_message")) -> ()  [unwired: 2 in, 2 out]
                          }
                          frame True {
                            n235 = flat-sequence {
                              tunnel: [w206] -> w198
                              tunnel: [w199] -> w196
                              tunnel: w198 -> [w213]
                              tunnel: [w213] -> w197
                              tunnel: w196 -> [w211]
                              tunnel: w197 -> [w221]
                              frame #0 {
                                n236 = property on="indicator_move_index" class="DigNum (strict)"() -> ("Value"=w209:dbl)  [unwired: 2 in, 2 out]
                                n237 = property on="indicator_sequence_distance_x" class="DigNum (strict)"() -> ("Value"=w199:dbl)  [unwired: 2 in, 2 out]
                                n238 = Increment(x=w209) -> (x+1=w205:dbl)
                                n239 = property on="indicator_move_index" class="DigNum (strict)"("Value"=w205) -> ()  [unwired: 2 in, 2 out]
                                n240 = Multiply(x=i16 200, y=w205) -> (x*y=w204:dbl)
                                n241 = Multiply(x=w204, y=20000.0) -> (x*y=w202:dbl)
                                n242 = Multiply(x=w199, y=1000000.0) -> (x*y=w201:dbl)
                                n243 = Absolute Value(x=w201) -> (abs(x)=w200:dbl)
                                n244 = Greater Or Equal?(x=w202, y=w200) -> (x >= y?=w206:bool)
                              }
                              frame #1 {
                                n245 = Less Than 0?(x=w211) -> (x < 0?=w212:bool)
                                n246 = case shown="False" w212 {
                                tunnel: [i64 20000 ("index") i64 -20000 ("index")] -> w210
                                frame False {
                                }
                                frame True {
                                }
                                }
                                n247 = property on="indicator_devices_reference" class="Clust (strict)"() -> ("Value"=w215:T11)  [unwired: 2 in, 2 out]
                                n248 = Unbundle By Name(w215) -> ("indicator_positioner_reference"=w214:refnum<class "SA_CTL.lvclass">)
                                n249 = call "Positioner Control.vi"("control_positioner_reference"=w214, "mode"="Incremental", "index"=w210, "control_move_direction"="x", "control_request"="Write") -> ()  [unwired: 1 in, 6 out]
                              }
                              frame #2 {
                                n250 = case shown="True" w221 {
                                frame False {
                                }
                                frame True {
                                n251 = property on="indicator_move_index" class="DigNum (strict)"("Val(Sgnl)"=i16 0 ("Value (Signaling)")) -> ()  [unwired: 2 in, 2 out]
                                n252 = property on="indicator_message" class="Str"("Value"="Moving stage y" ("indicator_message")) -> ()  [unwired: 2 in, 2 out]
                                }
                                }
                              }
                            }
                          }
                        }
                      }
                    }
                  }
                  frame "Stage x moved" {
                    n253 = property on="indicator_devices_reference" class="Clust (strict)"() -> ("Value"=w226:T11)  [unwired: 2 in, 2 out]
                    n254 = Unbundle By Name(w226) -> ("indicator_positioner_reference"=w225:refnum<class "SA_CTL.lvclass">)
                    n255 = call "Positioner Control.vi"("control_positioner_reference"=w225, "control_request"="Is Moving") -> ("indicator_positioner_ismoving_x"=w224:bool)  [unwired: 4 in, 5 out]
                    n256 = case shown="False" w224 {
                      frame False {
                        n257 = property on="indicator_message" class="Str"("Value"="Moving stage y" ("indicator_message")) -> ()  [unwired: 2 in, 2 out]
                      }
                      frame True {
                      }
                    }
                  }
                  frame "Moving stage y" {
                    n258 = property on="indicator_sequence_move_y" class="Bool (strict)"() -> ("Value"=w229:bool)  [unwired: 2 in, 2 out]
                    n259 = case shown="True" w229 {
                      frame False {
                        n260 = property on="indicator_message" class="Str"("Value"="Stabilizing" ("indicator_message")) -> ()  [unwired: 2 in, 2 out]
                      }
                      frame True {
                        n261 = flat-sequence {
                          tunnel: [w241] -> w233
                          tunnel: [w234] -> w231
                          tunnel: w233 -> [w248]
                          tunnel: [w248] -> w232
                          tunnel: w231 -> [w245]
                          tunnel: w232 -> [w256]
                          frame #0 {
                            n262 = property on="indicator_move_index" class="DigNum (strict)"() -> ("Value"=w244:dbl)  [unwired: 2 in, 2 out]
                            n263 = property on="indicator_sequence_distance_y" class="DigNum (strict)"() -> ("Value"=w234:dbl)  [unwired: 2 in, 2 out]
                            n264 = Increment(x=w244) -> (x+1=w240:dbl)
                            n265 = property on="indicator_move_index" class="DigNum (strict)"("Value"=w240) -> ()  [unwired: 2 in, 2 out]
                            n266 = Multiply(x=i16 200, y=w240) -> (x*y=w239:dbl)
                            n267 = Multiply(x=w234, y=1000000.0) -> (x*y=w236:dbl)
                            n268 = Multiply(x=w239, y=20000.0) -> (x*y=w237:dbl)
                            n269 = Absolute Value(x=w236) -> (abs(x)=w235:dbl)
                            n270 = Greater Or Equal?(x=w237, y=w235) -> (x >= y?=w241:bool)
                          }
                          frame #1 {
                            n271 = Less Than 0?(x=w245) -> (x < 0?=w247:bool)
                            n272 = case shown="False" w247 {
                              tunnel: [i64 20000 ("index") i64 -20000 ("index")] -> w246
                              frame False {
                              }
                              frame True {
                              }
                            }
                            n273 = property on="indicator_devices_reference" class="Clust (strict)"() -> ("Value"=w250:T11)  [unwired: 2 in, 2 out]
                            n274 = Unbundle By Name(w250) -> ("indicator_positioner_reference"=w249:refnum<class "SA_CTL.lvclass">)
                            n275 = call "Positioner Control.vi"("control_positioner_reference"=w249, "mode"="Incremental", "index"=w246, "control_move_direction"="y", "control_request"="Write") -> ()  [unwired: 1 in, 6 out]
                          }
                          frame #2 {
                            n276 = case shown="True" w256 {
                              frame False {
                              }
                              frame True {
                                n277 = property on="indicator_message" class="Str"("Value"="Stabilizing" ("indicator_message")) -> ()  [unwired: 2 in, 2 out]
                              }
                            }
                          }
                        }
                      }
                    }
                  }
                  frame "Stage y moved" {
                    n278 = property on="indicator_devices_reference" class="Clust (strict)"() -> ("Value"=w260:T11)  [unwired: 2 in, 2 out]
                    n279 = Unbundle By Name(w260) -> ("indicator_positioner_reference"=w259:refnum<class "SA_CTL.lvclass">)
                    n280 = call "Positioner Control.vi"("control_positioner_reference"=w259, "control_request"="Is Moving") -> ("indicator_positioner_ismoving_y"=w258:bool)  [unwired: 4 in, 5 out]
                    n281 = case shown="False" w258 {
                      frame False {
                        n282 = property on="indicator_message" class="Str"("Value"="Stabilizing" ("indicator_message")) -> ()  [unwired: 2 in, 2 out]
                      }
                      frame True {
                      }
                    }
                  }
                  frame "Stabilizing" {
                    n283 = property on="indicator_error" class="DigNum (strict)"() -> ("Value"=w266:i16)  [unwired: 2 in, 2 out]
                    n284 = property on="indicator_detector_intensity" class="Str"() -> ("Value"=w265:string)  [unwired: 2 in, 2 out]
                    n285 = Equal?(x=w265, y="Unfocused") -> (x = y?=w263:bool)
                    n286 = Absolute Value(x=w266) -> (abs(x)=w267:i16)
                    n287 = case shown="True" w263 {
                      frame False {
                      }
                      frame True {
                        n288 = property on="indicator_message" class="Str"("Val(Sgnl)"="Ready" ("Value (Signaling)")) -> ()  [unwired: 2 in, 2 out]
                      }
                    }
                    n289 = Less?(x=w267, y=i16 50) -> (x < y?=w268:bool)
                    n290 = case shown="True" w268 {
                      frame False {
                      }
                      frame True {
                        n291 = property on="indicator_message" class="Str"("Value"="Starting acquisition" ("indicator_message")) -> ()  [unwired: 2 in, 2 out]
                      }
                    }
                  }
                  frame "Starting acquisition" {
                    n292 = property on="indicator_sequence_current_parameters" class="Clust (strict)"() -> ("Value"=w283:T3)  [unwired: 2 in, 2 out]
                    n293 = property on="indicator_sequence_parameters" class="Clust (strict)"() -> ("Value"=w280:T4)  [unwired: 2 in, 2 out]
                    n294 = property on="indicator_sequence_parameters" class="Clust (strict)"() -> ("Value"=w284:T4)  [unwired: 2 in, 2 out]
                    n295 = Unbundle By Name(w283) -> ("currentLaser"=w287:i32, "currentXWell"=w276:i32, "currentYWell"=w275:i32, "currentXFOV"=w274:i32, "currentYFOV"=w273:i32, "currentRepeat"=w272:i32)
                    n296 = Unbundle By Name(w280) -> ("frames"=w279:i32[][])
                    n297 = Unbundle By Name(w284) -> ("lasers"=w285:string[][])
                    n298 = Decrement(x=w287) -> (x-1=w281:i32)
                    n299 = Index Array(array=w279, index (row)=0, index (col)=w281) -> (element=w277:i32)
                    n300 = Index Array(array=w285, index (row)=0, index (col)=w281) -> (element=w278:string)
                    n301 = stacked-sequence {
                      tunnel: w278 -> [w288 w300 _ w325 _]
                      tunnel: w277 -> [_ _ w318 _ _]
                      tunnel: w276 -> [_ _ _ w330 _]
                      tunnel: w275 -> [_ _ _ w329 _]
                      tunnel: w274 -> [_ _ _ w328 _]
                      tunnel: w273 -> [_ _ _ w327 _]
                      tunnel: w272 -> [_ _ _ w326 _]
                      frame #0 {
                        n302 = stacked-sequence {
                          tunnel: w288 -> [w289 _ w293]
                          frame #0 {
                            n303 = property on="indicator_light_source" class="Str"("Val(Sgnl)"=w289) -> ()  [unwired: 2 in, 2 out]
                            n304 = property on="indicator_current_filter_index" class="DigNum (strict)"() -> ("Value"=w290:u64)  [unwired: 2 in, 2 out]
                            n305 = call "Filter Control.vi"("control_current_filter_index"=w290, "control_laser_source"=w289, "control_request"="Write") -> ()  [unwired: 8 in, 1 out]
                          }
                          frame #1 {
                            n306 = Wait (ms)(milliseconds to wait=u32 1000) -> ()  [unwired: 1 out]
                          }
                          frame #2 {
                            n307 = case shown="\"Green\"" w293 {
                              tunnel: [u64 0 ("Value (Signaling)") u64 3 ("Value (Signaling)") u64 1 ("Value (Signaling)") u64 2 ("Value (Signaling)") u64 2 ("Value (Signaling)")] -> w294
                              frame "Red", Default {
                              }
                              frame "LED" {
                              }
                              frame "Green" {
                              }
                              frame "Blue" {
                              }
                              frame "Violet" {
                              }
                            }
                            n308 = property on="indicator_current_filter_index" class="DigNum (strict)"("Val(Sgnl)"=w294) -> ()  [unwired: 2 in, 2 out]
                          }
                        }
                      }
                      frame #1 {
                        n309 = case shown="\"LED\"" w300 {
                          tunnel: [w312 w313 w314 w315 u64 0 ("Value") w317] -> w310
                          frame "Blue" {
                            n310 = property on="indicator_blue_laser_power" class="DigNum (strict)"() -> ("Value"=w312:u64)  [unwired: 2 in, 2 out]
                          }
                          frame "Green" {
                            n311 = property on="indicator_green_laser_power" class="DigNum (strict)"() -> ("Value"=w313:u64)  [unwired: 2 in, 2 out]
                          }
                          frame "Red" {
                            n312 = property on="indicator_red_laser_power" class="DigNum (strict)"() -> ("Value"=w314:u64)  [unwired: 2 in, 2 out]
                          }
                          frame "LED" {
                            n313 = property on="indicator_LED_power" class="DigNum (strict)"() -> ("Value"=w315:u64)  [unwired: 2 in, 2 out]
                          }
                          frame Default {
                          }
                          frame "Violet" {
                            n314 = property on="indicator_violet_laser_power" class="DigNum (strict)"() -> ("Value"=w317:u64)  [unwired: 2 in, 2 out]
                          }
                        }
                        n315 = property on="indicator_devices_reference" class="Clust (strict)"() -> ("Value"=w307:T11)  [unwired: 2 in, 2 out]
                        n316 = Unbundle By Name(w307) -> ("indicator_light_source_channel_0_reference"=w302:u64, "indicator_light_source_channel_1_reference"=w303:u64, "indicator_light_source_channel_2_reference"=w304:u64, "indicator_light_source_channel_3_reference"=w305:u64, "indicator_light_source_LED_reference"=w306:u64, "indicator_light_source_LED_reference 2"=w301:u64)
                        n317 = Divide(x=w310, y=u64 100) -> (x/y=w308:dbl)
                        n318 = call "Laser Control.vi"("control_laser_source_channel_0_reference"=w302, "control_laser_source_LED_reference"=w301, "control_request"="Write", "control_laser_source_channel_1_reference"=w303, "control_laser_source_channel_2_reference"=w304, "control_laser_source_channel_3_reference"=w305, "control_laser_source_vibrator_reference"=w306, "control_laser_source"=w300, "control_laser_source_power"=w308) -> ()  [unwired: 7 out]
                      }
                      frame #2 {
                        n319 = property on="indicator_devices_reference" class="Clust (strict)"() -> ("Value"=w321:T11)  [unwired: 2 in, 2 out]
                        n320 = property on="control_exposure" class="Str"() -> ("Value"=w322:string)  [unwired: 2 in, 2 out]
                        n321 = Unbundle By Name(w321) -> ("indicator_library_reference"=w320:refnum<k24>, "indicator_camera_reference"=w319:refnum<k24>)  [unwired: 4 out]
                        n322 = Decimal String To Number(string=w322) -> (number=w323:i32)  [unwired: 2 in, 1 out]
                        n323 = call "Camera Control.vi"("control_camera_frames"=w318, "control_request"="Set", "control_camera_exposure_time"=w323, "control_library_reference"=w320, "control_camera_reference"=w319) -> ()  [unwired: 6 in, 5 out]
                      }
                      frame #3 {
                        n324 = stacked-sequence {
                          seq-local: [w337 _ _] -> [_ w375 _]
                          seq-local: [_ w375 _] -> [_ _ w379]
                          tunnel: w330 -> [w336 _ _]
                          tunnel: w329 -> [w335 _ _]
                          tunnel: w328 -> [w334 _ _]
                          tunnel: w327 -> [w333 _ _]
                          tunnel: w326 -> [w332 _ _]
                          tunnel: w325 -> [w331 _ _]
                          frame #0 {
                            n325 = property on="control_saving_path" class="Path"() -> ("Value"=w341:path)  [unwired: 2 in, 2 out]
                            n326 = property on="control_sequence" class="Bool (strict)"() -> ("Value"=w338:bool)  [unwired: 2 in, 2 out]
                            n327 = case shown="True" w338 {
                              tunnel: w341 -> [w347 w362]
                              tunnel: [w348 w359] -> w337
                              tunnel: w336 -> [_ w354]
                              tunnel: w335 -> [_ w353]
                              tunnel: w334 -> [_ w352]
                              tunnel: w333 -> [_ w351]
                              tunnel: w332 -> [_ w350]
                              tunnel: w331 -> [_ w349]
                              frame False {
                                n328 = property on="indicator_current_folder" class="DigNum (strict)"() -> ("Value"=w344:u64)  [unwired: 2 in, 2 out]
                                n329 = Increment(x=w344) -> (x+1=w342:u64)
                                n330 = property on="indicator_current_folder" class="DigNum (strict)"("Val(Sgnl)"=w342) -> ()  [unwired: 2 in, 2 out]
                                n331 = Path To String(path=w347) -> (string=w346:string)
                                n332 = Number To Decimal String(number=w342) -> (decimal integer string=w343:string)  [unwired: 1 in]
                                n333 = Concatenate Strings(w346, "\\" ("string"), w343) -> (w348:string)
                              }
                              frame True {
                                n334 = Path To String(path=w362) -> (string=w360:string)
                                n335 = Number To Decimal String(number=w354) -> (decimal integer string=w364:string)  [unwired: 1 in]
                                n336 = Number To Decimal String(number=w353) -> (decimal integer string=w366:string)  [unwired: 1 in]
                                n337 = Number To Decimal String(number=w352) -> (decimal integer string=w368:string)  [unwired: 1 in]
                                n338 = Number To Decimal String(number=w351) -> (decimal integer string=w370:string)  [unwired: 1 in]
                                n339 = Number To Decimal String(number=w350) -> (decimal integer string=w373:string)  [unwired: 1 in]
                                n340 = Concatenate Strings(w360, "\\" ("string"), w349, "_" ("string"), "xwell" ("string"), w364, "_" ("string"), "ywell" ("string"), w366, "_" ("string"), "xfov" ("string"), w368, "_" ("string"), "yfov" ("string"), w370, "_" ("string"), "repeat" ("string"), w373) -> (w359:string)
                              }
                            }
                            n341 = property on="indicator_folder_path" class="Str"("Val(Sgnl)"=w337) -> ()  [unwired: 2 in, 2 out]
                            n342 = String To Path(string=w337) -> (path=w340:path)
                            n343 = Create Folder(path (use dialog)=w340) -> (error out=→"error out 2":errorcluster)  [unwired: 2 in, 2 out]
                          }
                          frame #1 {
                            n344 = Wait (ms)(milliseconds to wait=u32 1000) -> ()  [unwired: 1 out]
                          }
                          frame #2 {
                            n345 = property on="indicator_devices_reference" class="Clust (strict)"() -> ("Value"=w378:T11)  [unwired: 2 in, 2 out]
                            n346 = Unbundle By Name(w378) -> ("indicator_library_reference"=w377:refnum<k24>, "indicator_camera_reference"=w376:refnum<k24>)
                            n347 = call "Camera Control.vi"("control_saving_file_path"=w379, "control_request"="Acquire", "control_library_reference"=w377, "control_camera_reference"=w376) -> ()  [unwired: 7 in, 5 out]
                          }
                        }
                      }
                      frame #4 {
                        n348 = Tick Count (ms)() -> (millisecond timer value=w383:u32)
                        n349 = Divide(x=w383, y=u32 1000) -> (x/y=w381:dbl)
                        n350 = property on="indicator_message" class="Str"("Val(Sgnl)"="Acquiring" ("Value (Signaling)")) -> ()  [unwired: 2 in, 2 out]
                        n351 = property on="indicator_acquisition_start_time" class="DigNum (strict)"("Val(Sgnl)"=w381) -> ()  [unwired: 2 in, 2 out]
                      }
                    }
                  }
                  frame "Default", Default {
                  }
                  frame "Initiating acquisition" {
                    # "Initiating / Setting Acquisition"
                    n352 = stacked-sequence {
                      frame #0 {
                        n353 = property on="control_sequence" class="Bool (strict)"() -> ("Value"=w385:bool)  [unwired: 2 in, 2 out]
                        n354 = case shown="True" w385 {
                          frame False {
                            w388 = 1 ("numXWells")
                            w389 = 0 ("distXWell")
                            w390 = 1 ("currentRepeat")
                            w398 = 1 ("dimension size")
                            w401 = 1 ("dimension size")
                            w402 = 0 ("distXWell")
                            n355 = property on="indicator_UV_activation_intensity" class="DigNum (strict)"("Val(Sgnl)"=0.0 ("Value (Signaling)")) -> ()  [unwired: 2 in, 2 out]
                            n356 = property on="indicator_UV_activation_time" class="DigNum (strict)"("Val(Sgnl)"=1000.0 ("Value (Signaling)")) -> ()  [unwired: 2 in, 2 out]
                            n357 = property on="control_frames" class="Str"() -> ("Value"=w392:string)  [unwired: 2 in, 2 out]
                            n358 = property on="indicator_light_source" class="Str"() -> ("Value"=w391:string)  [unwired: 2 in, 2 out]
                            n359 = property on="indicator_sequence_parameters" class="Clust (strict)"() -> ("Value"=w395:T4)  [unwired: 2 in, 2 out]
                            n360 = Decimal String To Number(string=w392) -> (number=w400:i32)  [unwired: 2 in, 1 out]
                            n361 = Initialize Array(w391, w398, w398) -> (w397:string[][])
                            n362 = Initialize Array(w400, w401, w401) -> (w399:i32[][])
                            n363 = Bundle By Name(cluster=w395, "numXWells"=w388, "numYWells"=w388, "numXFOVs"=w388, "numYFOVs"=w388, "numRepeats"=w388, "numLasers"=w388, "distXWell"=w402, "distYWell"=w402, "distXFOV"=w402, "distYFOV"=w402, "frames"=w399, "lasers"=w397) -> (w394:T4)
                            n364 = property on="indicator_sequence_current_parameters" class="Clust (strict)"() -> ("Value"=w396:T3)  [unwired: 2 in, 2 out]
                            n365 = property on="indicator_sequence_parameters" class="Clust (strict)"("Val(Sgnl)"=w394) -> ()  [unwired: 2 in, 2 out]
                            n366 = Bundle By Name(cluster=w396, "currentRepeat"=w390, "currentXWell"=w390, "currentYWell"=w390, "currentXFOV"=w390, "currentYFOV"=w390, "currentLaser"=w390, "distXWell"=w389, "distYWell"=w389, "distXFOV"=w389, "distYFOV"=w389) -> (w393:T3)
                            n367 = property on="indicator_sequence_current_parameters" class="Clust (strict)"("Val(Sgnl)"=w393) -> ()  [unwired: 2 in, 2 out]
                          }
                          frame True {
                            n368 = property on="indicator_saved_positions" class="Arr (strict)"() -> ("Value"=w403:i64[][])  [unwired: 2 in, 2 out]
                            n369 = Array Size(array=w403) -> (size(s)=w408:i32[])
                            n370 = Index Array(array=w408, index=0) -> (element=w404:i32)
                            n371 = Greater Than 0?(x=w404) -> (x > 0?=w406:bool)
                            n372 = case shown="True" w406 {
                              tunnel: [w410 w437] -> w409
                              tunnel: [w411 w432] -> w405
                              tunnel: w404 -> [_ w434]
                              tunnel: w403 -> [_ w422]
                              frame False {
                                n373 = property on="indicator_sequence_current_parameters" class="Clust (strict)"() -> ("Value"=w411:T3)  [unwired: 2 in, 2 out]
                                n374 = property on="indicator_sequence_parameters" class="Clust (strict)"() -> ("Value"=w410:T4)  [unwired: 2 in, 2 out]
                              }
                              frame True {
                                w412 = TRUE ("Value (Signaling)")
                                w415 = 1000000.0 ("y")
                                w430 = 0 ("distXFOV")
                                w435 = 0 ("distXFOV")
                                w433 = 1 ("numXWells")
                                n375 = Index Array(array=w422, index (row)=0 ("disabled index (row)"), index (col)=0 ("disabled index (col)")) -> (element=w418:i64)
                                n376 = Index Array(array=w422, index (row)=0 ("disabled index (row)"), index (col)=1 ("disabled index (col)")) -> (element=w419:i64)
                                n377 = property on="indicator_sequence_move_x" class="Bool (strict)"("Val(Sgnl)"=w412) -> ()  [unwired: 2 in, 2 out]
                                n378 = property on="indicator_sequence_move_y" class="Bool (strict)"("Val(Sgnl)"=w412) -> ()  [unwired: 2 in, 2 out]
                                n379 = property on="indicator_positioner_current_position" class="Arr (strict)"() -> ("Value"=w428:i64[])  [unwired: 2 in, 2 out]
                                n380 = Index Array(array=w428, index=0) -> (element=w426:i64)
                                n381 = Index Array(array=w428, index=1) -> (element=w425:i64)
                                n382 = Subtract(x=w418, y=w426) -> (x-y=w414:i64)
                                n383 = Subtract(x=w419, y=w425) -> (x-y=w413:i64)
                                n384 = property on="indicator_sequence_parameters" class="Clust (strict)"() -> ("Value"=w436:T4)  [unwired: 2 in, 2 out]
                                n385 = Divide(x=w414, y=w415) -> (x/y=w417:dbl)
                                n386 = Divide(x=w413, y=w415) -> (x/y=w416:dbl)
                                n387 = property on="indicator_sequence_current_parameters" class="Clust (strict)"() -> ("Value"=w431:T3)  [unwired: 2 in, 2 out]
                                n388 = property on="indicator_sequence_distance_x" class="DigNum (strict)"("Val(Sgnl)"=w417) -> ()  [unwired: 2 in, 2 out]
                                n389 = property on="indicator_sequence_distance_y" class="DigNum (strict)"("Val(Sgnl)"=w416) -> ()  [unwired: 2 in, 2 out]
                                n390 = Bundle By Name(cluster=w436, "numXWells"=w433, "numYWells"=w434, "numXFOVs"=w433, "numYFOVs"=w433, "distXWell"=w414, "distYWell"=w413, "distXFOV"=w435, "distYFOV"=w435) -> (w437:T4)
                                n391 = Bundle By Name(cluster=w431, "distXWell"=w414, "distYWell"=w413, "distXFOV"=w430, "distYFOV"=w430) -> (w432:T3)
                              }
                            }
                            n392 = property on="indicator_sequence_parameters" class="Clust (strict)"("Val(Sgnl)"=w409) -> ()  [unwired: 2 in, 2 out]
                            n393 = property on="indicator_sequence_current_parameters" class="Clust (strict)"("Val(Sgnl)"=w405) -> ()  [unwired: 2 in, 2 out]
                          }
                        }
                      }
                      frame #1 {
                        n394 = property on="indicator_message" class="Str"("Val(Sgnl)"="Setting acquisition" ("Value (Signaling)")) -> ()  [unwired: 2 in, 2 out]
                      }
                    }
                  }
                }
                n395 = property on="indicator_control_sequence" class="Bool (strict)"() -> ("Value"=w95:bool)  [unwired: 2 in, 2 out]
                n396 = property on="indicator_devices_reference" class="Clust (strict)"() -> ("Value"=w183:T11)  [unwired: 2 in, 2 out]
                n397 = property on="indicator_joystick_buttons" class="Clust (strict)"() -> ("Value"=w180:T7)  [unwired: 2 in, 2 out]
                n398 = property on="indicator_focus_status" class="Str"() -> ("Value"=w123:string)  [unwired: 2 in, 2 out]
                n399 = Unbundle By Name(w125) -> ("y"=w92:i16, "sum"=w89:u16)  [unwired: 1 out]
                n400 = property on="indicator_focus_status" class="Str"() -> ("Value"=w119:string)  [unwired: 2 in, 2 out]
                n401 = Unbundle By Name(w180) -> ("Square"=w177:bool, "X"=w176:bool, "Circle"=w178:bool, "Triangle"=w175:bool, "R1"=w105:bool, "R2"=w102:bool, "Playstation Button"=w179:bool, "Pad"=w140:bool, "L1"=w104:bool, "L2"=w103:bool)
                n402 = property on="indicator_sequence_current_parameters" class="Clust (strict)"() -> ("Value"=w171:T3)  [unwired: 2 in, 2 out]
                n403 = property on="control_sequence" class="Bool (strict)"() -> ("Value"=w94:bool)  [unwired: 2 in, 2 out]
                n404 = Greater?(x=w89, y=10000.0) -> (0:w120:bool)
                n405 = Not(x=w95) -> (.not. x?=w96:bool)
                n406 = Absolute Value(x=w130) -> (abs(x)=w132:i32)
                n407 = Absolute Value(x=w127) -> (abs(x)=w128:i32)
                n408 = Absolute Value(x=w134) -> (abs(x)=w135:i32)
                n409 = Absolute Value(x=w131) -> (abs(x)=w133:i32)
                n410 = call "Positioner Control.vi"("control_positioner_reference"=w112, "control_request"="Read") -> ("indicator_positioner_position"=w110:cluster{"x":i64, "y":i64, "z":i64})  [unwired: 4 in, 5 out]
                n411 = call "Joystick Control.vi"("control_request"="Read", "control_devices_reference"=w183) -> ("indicatror_joystick_axes"=w181:T5, "indicator_joystick_buttons"=w182:T7)  [unwired: 5 in, 3 out]
                n412 = property on="indicator_sequence_parameters" class="Clust (strict)"() -> ("Value"=w172:T4)  [unwired: 2 in, 2 out]
                n413 = Number To Fractional String(number=w89, precision (6)=i16 0) -> (F-format string=w99:string)  [unwired: 2 in]
                n414 = Equal?(x=w123, y="Locked") -> (x = y?=w121:bool)
                n415 = property on="indicator_detector_intensity" class="Str"("Val(Sgnl)"=w99) -> ()  [unwired: 2 in, 2 out]
                n416 = case shown="True" w179 {
                  frame False {
                  }
                  frame True {
                    # "Toggles Focus Status Indicator to 'Locked' if 'Focused' and Vice Versa as Well as Registers the 'Lock' Button Pressed."
                    n417 = stacked-sequence {
                      frame #0 {
                        n418 = property on="indicator_focus_status" class="Str"() -> ("Value"=w975:string)  [unwired: 2 in, 2 out]
                        n419 = case shown="\"Locked\"" w975 {
                          frame "Focused" {
                            n420 = property on="indicator_focus_userlocked" class="Bool (strict)"("Val(Sgnl)"=TRUE) -> ()  [unwired: 2 in, 2 out]
                            n421 = property on="indicator_focus_status" class="Str"("Val(Sgnl)"="Locked" ("Value (Signaling)")) -> ()  [unwired: 2 in, 2 out]
                          }
                          frame "Unfocused" {
                            n422 = property on="indicator_focus_userlocked" class="Bool (strict)"("Val(Sgnl)"=FALSE ("Value (Signaling)")) -> ()  [unwired: 2 in, 2 out]
                          }
                          frame "Default", Default {
                          }
                          frame "Locked" {
                            n423 = property on="indicator_focus_userlocked" class="Bool (strict)"("Val(Sgnl)"=FALSE ("Value (Signaling)")) -> ()  [unwired: 2 in, 2 out]
                            n424 = property on="indicator_focus_status" class="Str"("Val(Sgnl)"="Focused" ("Value (Signaling)")) -> ()  [unwired: 2 in, 2 out]
                          }
                        }
                      }
                      frame #1 {
                        n425 = property on="Playstation Button" class="Bool (strict)"("Val(Sgnl)"=FALSE ("Value (Signaling)")) -> ()  [unwired: 2 in, 2 out]
                      }
                      frame #2 {
                        n426 = Wait (ms)(milliseconds to wait=u32 1000) -> ()  [unwired: 1 out]
                      }
                    }
                  }
                }
                n427 = stacked-sequence {
                  seq-local: [w713 _ _] -> [_ w743 _]
                  seq-local: [w712 _ _] -> [_ w742 _]
                  seq-local: [w711 _ _] -> [_ w741 _]
                  seq-local: [w710 _ _] -> [_ w740 _]
                  seq-local: [w702 _ _] -> [_ w739 _]
                  seq-local: [_ w743 _] -> [_ _ w794]
                  seq-local: [_ w742 _] -> [_ _ w793]
                  seq-local: [_ w741 _] -> [_ _ w792]
                  seq-local: [_ w740 _] -> [_ _ w791]
                  seq-local: [_ w739 _] -> [_ _ w790]
                  tunnel: w177 -> [w717 _ _]
                  tunnel: w176 -> [w716 _ _]
                  tunnel: w178 -> [w715 _ _]
                  tunnel: w175 -> [w714 _ _]
                  tunnel: w140 -> [w703 _ _]
                  frame #0 {
                    # "Changes Light Source and Emission Filter Corresponding to the Button Pressed on the Joystick"
                    n428 = case shown="True" w717 {
                      tunnel: [FALSE TRUE] -> w713
                      frame False {
                      }
                      frame True {
                        n429 = property on="indicator_light_source" class="Str"("Val(Sgnl)"="Violet" ("Violet")) -> ()  [unwired: 2 in, 2 out]
                      }
                    }
                    n430 = case shown="True" w716 {
                      tunnel: [FALSE TRUE] -> w712
                      frame False {
                      }
                      frame True {
                        n431 = property on="indicator_light_source" class="Str"("Val(Sgnl)"="Blue" ("Value (Signaling)")) -> ()  [unwired: 2 in, 2 out]
                      }
                    }
                    n432 = case shown="True" w715 {
                      tunnel: [FALSE TRUE] -> w711
                      frame False {
                      }
                      frame True {
                        n433 = property on="indicator_light_source" class="Str"("Val(Sgnl)"="Red" ("Value (Signaling)")) -> ()  [unwired: 2 in, 2 out]
                      }
                    }
                    n434 = case shown="True" w714 {
                      tunnel: [FALSE TRUE] -> w710
                      frame False {
                      }
                      frame True {
                        n435 = property on="indicator_light_source" class="Str"("Val(Sgnl)"="Green" ("Value (Signaling)")) -> ()  [unwired: 2 in, 2 out]
                      }
                    }
                    n436 = case shown="True" w703 {
                      tunnel: [FALSE TRUE] -> w702
                      frame False {
                      }
                      frame True {
                        n437 = property on="indicator_light_source" class="Str"("Val(Sgnl)"="LED" ("Value (Signaling)")) -> ()  [unwired: 2 in, 2 out]
                      }
                    }
                    n438 = property on="indicator_light_source" class="Str"() -> ("Value"=w709:string)  [unwired: 2 in, 2 out]
                    n439 = case shown="\"LED\"" w709 {
                      tunnel: [w721 w722 w723 u64 0 ("Value") w725 w726] -> w708
                      frame "Blue" {
                        n440 = property on="indicator_blue_laser_power" class="DigNum (strict)"() -> ("Value"=w721:u64)  [unwired: 2 in, 2 out]
                      }
                      frame "Green" {
                        n441 = property on="indicator_green_laser_power" class="DigNum (strict)"() -> ("Value"=w722:u64)  [unwired: 2 in, 2 out]
                      }
                      frame "Red" {
                        n442 = property on="indicator_red_laser_power" class="DigNum (strict)"() -> ("Value"=w723:u64)  [unwired: 2 in, 2 out]
                      }
                      frame Default {
                      }
                      frame "LED" {
                        n443 = property on="indicator_LED_power" class="DigNum (strict)"() -> ("Value"=w725:u64)  [unwired: 2 in, 2 out]
                      }
                      frame "Violet" {
                        n444 = property on="indicator_violet_laser_power" class="DigNum (strict)"() -> ("Value"=w726:u64)  [unwired: 2 in, 2 out]
                      }
                    }
                    n445 = Divide(x=w708, y=u64 100) -> (x/y=w706:dbl)
                    n446 = Number To Fractional String(number=w706, precision (6)=i16 1) -> (F-format string=w705:string)  [unwired: 2 in]
                    n447 = property on="indicator_light_source_power" class="Str"("Val(Sgnl)"=w705) -> ()  [unwired: 2 in, 2 out]
                  }
                  frame #1 {
                    n448 = Build Array(w743, w742, w741, w740, w739) -> (w744:bool[])
                    n449 = Or Array Elements(Boolean array=w744) -> (logical OR=w745:bool)
                    n450 = case shown="True" w745 {
                      frame False {
                      }
                      frame True {
                        n451 = property on="indicator_light_source_power" class="Str"() -> ("Value"=w749:string)  [unwired: 2 in, 2 out]
                        n452 = property on="indicator_devices_reference" class="Clust (strict)"() -> ("Value"=w753:T11)  [unwired: 2 in, 2 out]
                        n453 = Unbundle By Name(w753) -> ("indicator_light_source_channel_0_reference"=w757:u64, "indicator_light_source_channel_1_reference"=w756:u64, "indicator_light_source_channel_2_reference"=w755:u64, "indicator_light_source_channel_3_reference"=w754:u64, "indicator_light_source_LED_reference"=w747:u64, "indicator_light_source_LED_reference 2"=w746:u64)
                        n454 = Decimal String To Number(string=w749) -> (number=w748:i32)  [unwired: 2 in, 1 out]
                        n455 = property on="indicator_current_filter_index" class="DigNum (strict)"() -> ("Value"=w750:u64)  [unwired: 2 in, 2 out]
                        n456 = property on="indicator_light_source" class="Str"() -> ("Value"=w751:string)  [unwired: 2 in, 2 out]
                        n457 = property on="indicator_message" class="Str"() -> ("Value"=w752:string)  [unwired: 2 in, 2 out]
                        n458 = case shown="\"Live\"" w752 {
                          tunnel: w757 -> [_ _ w769]
                          tunnel: w756 -> [_ _ w768]
                          tunnel: w755 -> [_ _ w767]
                          tunnel: w754 -> [_ _ w766]
                          tunnel: w751 -> [w759 _ w765]
                          tunnel: w750 -> [w758 _ w764]
                          tunnel: w748 -> [_ _ w763]
                          tunnel: w747 -> [_ _ w762]
                          tunnel: w746 -> [_ _ w761]
                          frame "Ready" {
                            n459 = call "Filter Control.vi"("control_current_filter_index"=w758, "control_laser_source"=w759, "control_request"="Write") -> ()  [unwired: 8 in, 1 out]
                          }
                          frame "Default", Default {
                          }
                          frame "Live" {
                            n460 = stacked-sequence {
                              tunnel: w769 -> [w776 _ w788]
                              tunnel: w768 -> [w775 _ w787]
                              tunnel: w767 -> [w773 _ w784]
                              tunnel: w766 -> [w772 _ w783]
                              tunnel: w765 -> [_ w779 w786]
                              tunnel: w764 -> [_ w778 _]
                              tunnel: w763 -> [_ _ w785]
                              tunnel: w762 -> [w771 _ w782]
                              tunnel: w761 -> [w770 _ w781]
                              frame #0 {
                                n461 = call "Laser Control.vi"("control_laser_source_channel_0_reference"=w776, "control_laser_source_LED_reference"=w770, "control_request"="Write", "control_laser_source_channel_1_reference"=w775, "control_laser_source_channel_2_reference"=w773, "control_laser_source_channel_3_reference"=w772, "control_laser_source_vibrator_reference"=w771, "control_laser_source"="None") -> ()  [unwired: 1 in, 7 out]
                              }
                              frame #1 {
                                n462 = call "Filter Control.vi"("control_current_filter_index"=w778, "control_laser_source"=w779, "control_request"="Write") -> ()  [unwired: 8 in, 1 out]
                              }
                              frame #2 {
                                n463 = call "Laser Control.vi"("control_laser_source_channel_0_reference"=w788, "control_laser_source_LED_reference"=w781, "control_request"="Write", "control_laser_source_channel_1_reference"=w787, "control_laser_source_channel_2_reference"=w784, "control_laser_source_channel_3_reference"=w783, "control_laser_source_vibrator_reference"=w782, "control_laser_source"=w786, "control_laser_source_power"=w785) -> ()  [unwired: 7 out]
                              }
                            }
                          }
                        }
                      }
                    }
                  }
                  frame #2 {
                    n464 = case shown="True" w794 {
                      frame False {
                        (unwired) FALSE
                      }
                      frame True {
                        n465 = property on="indicator_current_filter_index" class="DigNum (strict)"("Val(Sgnl)"=u64 2 ("Value (Signaling)")) -> ()  [unwired: 2 in, 2 out]
                      }
                    }
                    n466 = case shown="True" w793 {
                      frame False {
                        (unwired) FALSE
                      }
                      frame True {
                        n467 = property on="indicator_current_filter_index" class="DigNum (strict)"("Val(Sgnl)"=u64 2 ("Value (Signaling)")) -> ()  [unwired: 2 in, 2 out]
                      }
                    }
                    n468 = case shown="True" w792 {
                      frame False {
                        (unwired) FALSE
                      }
                      frame True {
                        n469 = property on="indicator_current_filter_index" class="DigNum (strict)"("Val(Sgnl)"=u64 0 ("Value (Signaling)")) -> ()  [unwired: 2 in, 2 out]
                      }
                    }
                    n470 = case shown="True" w791 {
                      frame False {
                        (unwired) FALSE
                      }
                      frame True {
                        n471 = property on="indicator_current_filter_index" class="DigNum (strict)"("Val(Sgnl)"=u64 1 ("Value (Signaling)")) -> ()  [unwired: 2 in, 2 out]
                      }
                    }
                    n472 = case shown="True" w790 {
                      frame False {
                        (unwired) FALSE
                      }
                      frame True {
                        n473 = property on="indicator_current_filter_index" class="DigNum (strict)"("Val(Sgnl)"=u64 3 ("Value (Signaling)")) -> ()  [unwired: 2 in, 2 out]
                      }
                    }
                  }
                }
                n474 = case shown="True" w105 {
                  frame False {
                  }
                  frame True {
                    # "Increasing the Power Level of the Selected Laser When the Corresponding Button is Pressed"
                    n475 = property on="indicator_light_source" class="Str"() -> ("Value"=w850:string)  [unwired: 2 in, 2 out]
                    n476 = case shown="\"LED\"" w850 {
                      tunnel: [w872 w873 w874 w875 u64 0 ("Value") w877] -> w856
                      frame "Blue" {
                        n477 = property on="indicator_blue_laser_power" class="DigNum (strict)"() -> ("Value"=w872:u64)  [unwired: 2 in, 2 out]
                      }
                      frame "Green" {
                        n478 = property on="indicator_green_laser_power" class="DigNum (strict)"() -> ("Value"=w873:u64)  [unwired: 2 in, 2 out]
                      }
                      frame "Red" {
                        n479 = property on="indicator_red_laser_power" class="DigNum (strict)"() -> ("Value"=w874:u64)  [unwired: 2 in, 2 out]
                      }
                      frame "LED" {
                        n480 = property on="indicator_LED_power" class="DigNum (strict)"() -> ("Value"=w875:u64)  [unwired: 2 in, 2 out]
                      }
                      frame Default {
                      }
                      frame "Violet" {
                        n481 = property on="indicator_violet_laser_power" class="DigNum (strict)"() -> ("Value"=w877:u64)  [unwired: 2 in, 2 out]
                      }
                    }
                    n482 = Add(x=w856, y=1.0) -> (x+y=w843:dbl)
                    n483 = In Range and Coerce(upper limit=500.0, x=w843, lower limit=0.0) -> (coerced(x)=w842:dbl)  [unwired: 1 out]
                    n484 = property on="indicator_devices_reference" class="Clust (strict)"() -> ("Value"=w849:T11)  [unwired: 2 in, 2 out]
                    n485 = Unbundle By Name(w849) -> ("indicator_light_source_channel_0_reference"=w848:u64, "indicator_light_source_channel_1_reference"=w847:u64, "indicator_light_source_channel_2_reference"=w846:u64, "indicator_light_source_channel_3_reference"=w845:u64, "indicator_light_source_LED_reference"=w840:u64, "indicator_light_source_LED_reference 2"=w839:u64)
                    n486 = case shown="\"LED\"" w850 {
                      tunnel: w842 -> [w867 w868 w869 w870 _ w871]
                      frame "Blue" {
                        n487 = property on="indicator_blue_laser_power" class="DigNum (strict)"("Val(Sgnl)"=w867) -> ()  [unwired: 2 in, 2 out]
                      }
                      frame "Green" {
                        n488 = property on="indicator_green_laser_power" class="DigNum (strict)"("Val(Sgnl)"=w868) -> ()  [unwired: 2 in, 2 out]
                      }
                      frame "Red" {
                        n489 = property on="indicator_red_laser_power" class="DigNum (strict)"("Val(Sgnl)"=w869) -> ()  [unwired: 2 in, 2 out]
                      }
                      frame "LED" {
                        n490 = property on="indicator_LED_power" class="DigNum (strict)"("Val(Sgnl)"=w870) -> ()  [unwired: 2 in, 2 out]
                      }
                      frame Default {
                      }
                      frame "Violet" {
                        n491 = property on="indicator_violet_laser_power" class="DigNum (strict)"("Val(Sgnl)"=w871) -> ()  [unwired: 2 in, 2 out]
                      }
                    }
                    n492 = property on="indicator_message" class="Str"() -> ("Value"=w851:string)  [unwired: 2 in, 2 out]
                    n493 = Divide(x=w842, y=100.0) -> (x/y=w844:dbl)
                    n494 = case shown="\"Live\"" w851 {
                      tunnel: w850 -> [_ w865]
                      tunnel: w848 -> [_ w864]
                      tunnel: w847 -> [_ w863]
                      tunnel: w846 -> [_ w861]
                      tunnel: w845 -> [_ w860]
                      tunnel: w844 -> [_ w862]
                      tunnel: w840 -> [_ w859]
                      tunnel: w839 -> [_ w858]
                      frame "Default", Default {
                      }
                      frame "Live" {
                        n495 = call "Laser Control.vi"("control_laser_source_channel_0_reference"=w864, "control_laser_source_LED_reference"=w858, "control_request"="Write", "control_laser_source_channel_1_reference"=w863, "control_laser_source_channel_2_reference"=w861, "control_laser_source_channel_3_reference"=w860, "control_laser_source_vibrator_reference"=w859, "control_laser_source"=w865, "control_laser_source_power"=w862) -> ()  [unwired: 7 out]
                      }
                    }
                    n496 = Number To Fractional String(number=w844, precision (6)=i16 1) -> (F-format string=w852:string)  [unwired: 2 in]
                    n497 = property on="indicator_light_source_power" class="Str"("Val(Sgnl)"=w852) -> ()  [unwired: 2 in, 2 out]
                  }
                }
                n498 = case shown="True" w102 {
                  frame False {
                  }
                  frame True {
                    # "Decreasing the Power Level of the Selected Laser When the Corresponding Button is Pressed"
                    n499 = property on="indicator_light_source" class="Str"() -> ("Value"=w810:string)  [unwired: 2 in, 2 out]
                    n500 = case shown="\"LED\"" w810 {
                      tunnel: [w833 w834 w835 w836 u64 0 ("Value") w838] -> w817
                      frame "Blue" {
                        n501 = property on="indicator_blue_laser_power" class="DigNum (strict)"() -> ("Value"=w833:u64)  [unwired: 2 in, 2 out]
                      }
                      frame "Green" {
                        n502 = property on="indicator_green_laser_power" class="DigNum (strict)"() -> ("Value"=w834:u64)  [unwired: 2 in, 2 out]
                      }
                      frame "Red" {
                        n503 = property on="indicator_red_laser_power" class="DigNum (strict)"() -> ("Value"=w835:u64)  [unwired: 2 in, 2 out]
                      }
                      frame "LED" {
                        n504 = property on="indicator_LED_power" class="DigNum (strict)"() -> ("Value"=w836:u64)  [unwired: 2 in, 2 out]
                      }
                      frame Default {
                      }
                      frame "Violet" {
                        n505 = property on="indicator_violet_laser_power" class="DigNum (strict)"() -> ("Value"=w838:u64)  [unwired: 2 in, 2 out]
                      }
                    }
                    n506 = Subtract(x=w817, y=1.0) -> (x-y=w803:dbl)
                    n507 = In Range and Coerce(upper limit=500.0, x=w803, lower limit=0.0) -> (coerced(x)=w813:dbl)  [unwired: 1 out]
                    n508 = property on="indicator_devices_reference" class="Clust (strict)"() -> ("Value"=w809:T11)  [unwired: 2 in, 2 out]
                    n509 = Unbundle By Name(w809) -> ("indicator_light_source_channel_0_reference"=w808:u64, "indicator_light_source_channel_1_reference"=w807:u64, "indicator_light_source_channel_2_reference"=w806:u64, "indicator_light_source_channel_3_reference"=w805:u64, "indicator_light_source_LED_reference"=w801:u64, "indicator_light_source_LED_reference 2"=w800:u64)
                    n510 = case shown="\"LED\"" w810 {
                      tunnel: w813 -> [w828 w829 w830 w831 _ w832]
                      frame "Blue" {
                        n511 = property on="indicator_blue_laser_power" class="DigNum (strict)"("Val(Sgnl)"=w828) -> ()  [unwired: 2 in, 2 out]
                      }
                      frame "Green" {
                        n512 = property on="indicator_green_laser_power" class="DigNum (strict)"("Val(Sgnl)"=w829) -> ()  [unwired: 2 in, 2 out]
                      }
                      frame "Red" {
                        n513 = property on="indicator_red_laser_power" class="DigNum (strict)"("Val(Sgnl)"=w830) -> ()  [unwired: 2 in, 2 out]
                      }
                      frame "LED" {
                        n514 = property on="indicator_LED_power" class="DigNum (strict)"("Val(Sgnl)"=w831) -> ()  [unwired: 2 in, 2 out]
                      }
                      frame Default {
                      }
                      frame "Violet" {
                        n515 = property on="indicator_violet_laser_power" class="DigNum (strict)"("Val(Sgnl)"=w832) -> ()  [unwired: 2 in, 2 out]
                      }
                    }
                    n516 = property on="indicator_message" class="Str"() -> ("Value"=w811:string)  [unwired: 2 in, 2 out]
                    n517 = Divide(x=w813, y=100.0) -> (x/y=w804:dbl)
                    n518 = case shown="\"Live\"" w811 {
                      tunnel: w810 -> [_ w826]
                      tunnel: w808 -> [_ w825]
                      tunnel: w807 -> [_ w824]
                      tunnel: w806 -> [_ w822]
                      tunnel: w805 -> [_ w821]
                      tunnel: w804 -> [_ w823]
                      tunnel: w801 -> [_ w820]
                      tunnel: w800 -> [_ w819]
                      frame "Default", Default {
                      }
                      frame "Live" {
                        n519 = call "Laser Control.vi"("control_laser_source_channel_0_reference"=w825, "control_laser_source_LED_reference"=w819, "control_request"="Write", "control_laser_source_channel_1_reference"=w824, "control_laser_source_channel_2_reference"=w822, "control_laser_source_channel_3_reference"=w821, "control_laser_source_vibrator_reference"=w820, "control_laser_source"=w826, "control_laser_source_power"=w823) -> ()  [unwired: 7 out]
                      }
                    }
                    n520 = Number To Fractional String(number=w804, precision (6)=i16 1) -> (F-format string=w812:string)  [unwired: 2 in]
                    n521 = property on="indicator_light_source_power" class="Str"("Val(Sgnl)"=w812) -> ()  [unwired: 2 in, 2 out]
                  }
                }
                n522 = case shown="True" w103 {
                  frame False {
                  }
                  frame True {
                    # "Initiating / Terminating Acquisition when the Corresponding Button is Pressed on the Joystick"
                    n523 = property on="indicator_message" class="Str"() -> ("Value"=w983:string)  [unwired: 2 in, 2 out]
                    n524 = case shown="\"Ready\"" w983 {
                      frame "Acquiring" {
                        n525 = property on="indicator_devices_reference" class="Clust (strict)"() -> ("Value"=w986:T11)  [unwired: 2 in, 2 out]
                        n526 = Unbundle By Name(w986) -> ("indicator_light_source_channel_0_reference"=w992:u64, "indicator_light_source_channel_1_reference"=w991:u64, "indicator_light_source_channel_2_reference"=w990:u64, "indicator_light_source_channel_3_reference"=w989:u64, "indicator_light_source_LED_reference"=w985:u64, "indicator_light_source_LED_reference 2"=w984:u64, "indicator_library_reference"=w988:refnum<k24>, "indicator_camera_reference"=w987:refnum<k24>)
                        n527 = stacked-sequence {
                          tunnel: w992 -> [w998 _ _ _ _]
                          tunnel: w991 -> [w997 _ _ _ _]
                          tunnel: w990 -> [w996 _ _ _ _]
                          tunnel: w989 -> [w995 _ _ _ _]
                          tunnel: w988 -> [_ w1002 _ _ _]
                          tunnel: w987 -> [_ w1001 _ _ _]
                          tunnel: w985 -> [w994 _ _ _ _]
                          tunnel: w984 -> [w993 _ _ _ _]
                          frame #0 {
                            n528 = call "Laser Control.vi"("control_laser_source_channel_0_reference"=w998, "control_laser_source_LED_reference"=w993, "control_request"="Write", "control_laser_source_channel_1_reference"=w997, "control_laser_source_channel_2_reference"=w996, "control_laser_source_channel_3_reference"=w995, "control_laser_source_vibrator_reference"=w994, "control_laser_source"="None") -> ()  [unwired: 1 in, 7 out]
                          }
                          frame #1 {
                            n529 = call "Camera Control.vi"("control_request"="Stop", "control_library_reference"=w1002, "control_camera_reference"=w1001) -> ()  [unwired: 8 in, 5 out]
                          }
                          frame #2 {
                            n530 = Wait (ms)(milliseconds to wait=u32 1000) -> ()  [unwired: 1 out]
                          }
                          frame #3 {
                            n531 = property on="indicator_joystick_buttons" class="Clust (strict)"() -> ("Value"=w1006:T7)  [unwired: 2 in, 2 out]
                            n532 = Bundle By Name(cluster=w1006, "L2"=FALSE ("R1")) -> (w1007:T7)
                            n533 = property on="indicator_joystick_buttons" class="Clust (strict)"("Val(Sgnl)"=w1007) -> ()  [unwired: 2 in, 2 out]
                          }
                          frame #4 {
                            n534 = property on="indicator_message" class="Str"("Val(Sgnl)"="Ready" ("Value (Signaling)")) -> ()  [unwired: 2 in, 2 out]
                          }
                        }
                      }
                      frame "Default", Default {
                      }
                      frame "Ready" {
                        n535 = property on="indicator_message" class="Str"("Val(Sgnl)"="Initiating acquisition" ("Value (Signaling)")) -> ()  [unwired: 2 in, 2 out]
                      }
                    }
                  }
                }
                n536 = case shown="True" w104 {
                  frame False {
                  }
                  frame True {
                    # "Initiating / Terminating Live Imaging when the Corresponding Button is Pressed on the Joystick"
                    n537 = property on="indicator_message" class="Str"() -> ("Value"=w1010:string)  [unwired: 2 in, 2 out]
                    n538 = case shown="\"Live\"" w1010 {
                      frame "Live" {
                        n539 = property on="indicator_devices_reference" class="Clust (strict)"() -> ("Value"=w1013:T11)  [unwired: 2 in, 2 out]
                        n540 = Unbundle By Name(w1013) -> ("indicator_light_source_channel_0_reference"=w1019:u64, "indicator_light_source_channel_1_reference"=w1018:u64, "indicator_light_source_channel_2_reference"=w1017:u64, "indicator_light_source_channel_3_reference"=w1016:u64, "indicator_light_source_LED_reference"=w1012:u64, "indicator_light_source_LED_reference 2"=w1011:u64, "indicator_library_reference"=w1015:refnum<k24>, "indicator_camera_reference"=w1014:refnum<k24>)
                        n541 = stacked-sequence {
                          tunnel: w1019 -> [w1025 _ _ _ _]
                          tunnel: w1018 -> [w1024 _ _ _ _]
                          tunnel: w1017 -> [w1023 _ _ _ _]
                          tunnel: w1016 -> [w1022 _ _ _ _]
                          tunnel: w1015 -> [_ w1029 _ _ _]
                          tunnel: w1014 -> [_ w1028 _ _ _]
                          tunnel: w1012 -> [w1021 _ _ _ _]
                          tunnel: w1011 -> [w1020 _ _ _ _]
                          frame #0 {
                            n542 = call "Laser Control.vi"("control_laser_source_channel_0_reference"=w1025, "control_laser_source_LED_reference"=w1020, "control_request"="Write", "control_laser_source_channel_1_reference"=w1024, "control_laser_source_channel_2_reference"=w1023, "control_laser_source_channel_3_reference"=w1022, "control_laser_source_vibrator_reference"=w1021, "control_laser_source"="None") -> ()  [unwired: 1 in, 7 out]
                          }
                          frame #1 {
                            n543 = call "Camera Control.vi"("control_request"="Stop", "control_library_reference"=w1029, "control_camera_reference"=w1028) -> ()  [unwired: 8 in, 5 out]
                          }
                          frame #2 {
                            n544 = Wait (ms)(milliseconds to wait=u32 1000) -> ()  [unwired: 1 out]
                          }
                          frame #3 {
                            n545 = property on="indicator_joystick_buttons" class="Clust (strict)"() -> ("Value"=w1033:T7)  [unwired: 2 in, 2 out]
                            n546 = Bundle By Name(cluster=w1033, "L1"=FALSE ("R1")) -> (w1034:T7)
                            n547 = property on="indicator_joystick_buttons" class="Clust (strict)"("Val(Sgnl)"=w1034) -> ()  [unwired: 2 in, 2 out]
                          }
                          frame #4 {
                            n548 = property on="indicator_message" class="Str"("Val(Sgnl)"="Ready" ("Value (Signaling)")) -> ()  [unwired: 2 in, 2 out]
                          }
                        }
                      }
                      frame "Default", Default {
                      }
                      frame "Ready" {
                        n549 = property on="indicator_devices_reference" class="Clust (strict)"() -> ("Value"=w1038:T11)  [unwired: 2 in, 2 out]
                        n550 = Unbundle By Name(w1038) -> ("indicator_light_source_channel_0_reference"=w1044:u64, "indicator_light_source_channel_1_reference"=w1043:u64, "indicator_light_source_channel_2_reference"=w1042:u64, "indicator_light_source_channel_3_reference"=w1041:u64, "indicator_light_source_LED_reference"=w1037:u64, "indicator_light_source_LED_reference 2"=w1036:u64, "indicator_library_reference"=w1040:refnum<k24>, "indicator_camera_reference"=w1039:refnum<k24>)
                        n551 = stacked-sequence {
                          tunnel: w1044 -> [_ w1056 _ _ _ _]
                          tunnel: w1043 -> [_ w1055 _ _ _ _]
                          tunnel: w1042 -> [_ w1051 _ _ _ _]
                          tunnel: w1041 -> [_ w1050 _ _ _ _]
                          tunnel: w1040 -> [_ _ w1062 w1064 _ _]
                          tunnel: w1039 -> [_ _ w1061 w1063 _ _]
                          tunnel: w1037 -> [_ w1049 _ _ _ _]
                          tunnel: w1036 -> [_ w1048 _ _ _ _]
                          frame #0 {
                            n552 = property on="indicator_current_filter_index" class="DigNum (strict)"() -> ("Value"=w1045:u64)  [unwired: 2 in, 2 out]
                            n553 = property on="indicator_light_source" class="Str"() -> ("Value"=w1046:string)  [unwired: 2 in, 2 out]
                            n554 = call "Filter Control.vi"("control_current_filter_index"=w1045, "control_laser_source"=w1046, "control_request"="Write") -> ()  [unwired: 8 in, 1 out]
                          }
                          frame #1 {
                            n555 = property on="indicator_light_source_power" class="Str"() -> ("Value"=w1053:string)  [unwired: 2 in, 2 out]
                            n556 = property on="indicator_light_source" class="Str"() -> ("Value"=w1054:string)  [unwired: 2 in, 2 out]
                            n557 = Decimal String To Number(string=w1053) -> (number=w1052:i32)  [unwired: 2 in, 1 out]
                            n558 = call "Laser Control.vi"("control_laser_source_channel_0_reference"=w1056, "control_laser_source_LED_reference"=w1048, "control_request"="Write", "control_laser_source_channel_1_reference"=w1055, "control_laser_source_channel_2_reference"=w1051, "control_laser_source_channel_3_reference"=w1050, "control_laser_source_vibrator_reference"=w1049, "control_laser_source"=w1054, "control_laser_source_power"=w1052) -> ()  [unwired: 7 out]
                          }
                          frame #2 {
                            n559 = property on="control_exposure" class="Str"() -> ("Value"=w1059:string)  [unwired: 2 in, 2 out]
                            n560 = Decimal String To Number(string=w1059) -> (number=w1058:i32)  [unwired: 2 in, 1 out]
                            n561 = call "Camera Control.vi"("control_request"="Set", "control_camera_exposure_time"=w1058, "control_library_reference"=w1062, "control_camera_reference"=w1061) -> ()  [unwired: 7 in, 5 out]
                          }
                          frame #3 {
                            n562 = call "Camera Control.vi"("control_request"="Live", "control_library_reference"=w1064, "control_camera_reference"=w1063) -> ()  [unwired: 8 in, 5 out]
                          }
                          frame #4 {
                            n563 = for {
                              N: 1000 -> [_]
                              n564 = property on="indicator_joystick_buttons" class="Clust (strict)"() -> ("Value"=w1068:T7)  [unwired: 2 in, 2 out]
                              n565 = Bundle By Name(cluster=w1068, "L1"=FALSE ("R1")) -> (w1069:T7)
                              n566 = property on="indicator_joystick_buttons" class="Clust (strict)"("Val(Sgnl)"=w1069) -> ()  [unwired: 2 in, 2 out]
                            }
                          }
                          frame #5 {
                            n567 = property on="indicator_message" class="Str"("Val(Sgnl)"="Live" ("Value (Signaling)")) -> ()  [unwired: 2 in, 2 out]
                          }
                        }
                      }
                    }
                  }
                }
                n568 = property on="indicator_positioner_reference" class="LVClassControl (strict)"() -> ("Value"=w101:refnum<class "SA_CTL.lvclass">)  [unwired: 2 in, 2 out]
                n569 = And(x=w94, y=w96) -> (x .and. y?=w97:bool)
                n570 = property on="indicator_devices_reference" class="Clust (strict)"() -> ("Value"=w150:T11)  [unwired: 2 in, 2 out]
                n571 = Greater?(x=w132, y=2000) -> (0:w114:bool)
                n572 = Greater?(x=w128, y=2000) -> (0:w117:bool)
                n573 = Greater?(x=w135, y=2000) -> (0:w91:bool)
                n574 = Greater?(x=w133, y=2000) -> (0:w90:bool)
                n575 = case shown="True" w97 {
                  tunnel: w94 -> [w459 _]
                  frame False {
                    n576 = case shown="False" w459 {
                      frame False {
                        n577 = property on="indicator_control_sequence" class="Bool (strict)"("Val(Sgnl)"=FALSE ("Value (Signaling)")) -> ()  [unwired: 2 in, 2 out]
                      }
                      frame True {
                      }
                    }
                  }
                  frame True {
                    n578 = stacked-sequence {
                      frame #0 {
                        n579 = property on="control_sequence_file_path" class="Path"() -> ("Value"=w461:path)  [unwired: 2 in, 2 out]
                        n580 = call "Sequence Module.vi"("control_request"="Read", "control_sequence_file_path"=w461) -> ("indicator_sequence_current_parameters"=w463:T3, "indicator_sequence_parameters"=w464:T4, "indicator_UV_activation_intensity"=w465:dbl, "indicator_UV_activation_time"=w466:dbl)  [unwired: 6 in, 4 out]
                        n581 = property on="indicator_sequence_current_parameters" class="Clust (strict)"("Val(Sgnl)"=w463) -> ()  [unwired: 2 in, 2 out]
                        n582 = property on="indicator_sequence_parameters" class="Clust (strict)"("Val(Sgnl)"=w464) -> ()  [unwired: 2 in, 2 out]
                        n583 = property on="indicator_UV_activation_intensity" class="DigNum (strict)"("Val(Sgnl)"=w465) -> ()  [unwired: 2 in, 2 out]
                        n584 = property on="indicator_UV_activation_time" class="DigNum (strict)"("Val(Sgnl)"=w466) -> ()  [unwired: 2 in, 2 out]
                      }
                      frame #1 {
                        n585 = property on="indicator_control_sequence" class="Bool (strict)"("Val(Sgnl)"=TRUE ("Value (Signaling)")) -> ()  [unwired: 2 in, 2 out]
                      }
                    }
                  }
                }
                n586 = case shown="False" w120 {
                  frame False {
                    n587 = property on="indicator_focus_status" class="Str"() -> ("Value"=w667:string)  [unwired: 2 in, 2 out]
                    n588 = Equal?(x=w667, y="Focused") -> (x = y?=w665:bool)
                    n589 = Equal?(x=w667, y="Locked") -> (x = y?=w664:bool)
                    n590 = Or(x=w665, y=w664) -> (x .or. y?=w663:bool)
                    n591 = case shown="True" w663 {
                      frame False {
                      }
                      frame True {
                        n592 = property on="indicator_focus_status" class="Str"("Val(Sgnl)"="Unfocused" ("Value (Signaling)")) -> ()  [unwired: 2 in, 2 out]
                      }
                    }
                  }
                  frame True {
                    # "Changing Focus Status Indicator to 'Unfocused', 'Focused' or 'Locked' Depending on the Intensity of the Returning IR Beam on the PSD and Whether the User has Pressed the 'Lock' (Playstation) Button"
                    n593 = property on="indicator_focus_status" class="Str"() -> ("Value"=w672:string)  [unwired: 2 in, 2 out]
                    n594 = Equal?(x=w672, y="Unfocused") -> (x = y?=w670:bool)
                    n595 = case shown="False" w670 {
                      frame False {
                      }
                      frame True {
                        n596 = property on="indicator_focus_userlocked" class="Bool (strict)"() -> ("Value"=w673:bool)  [unwired: 2 in, 2 out]
                        n597 = case shown="True" w673 {
                          tunnel: ["Focused" ("Value (Signaling)") "Locked" ("Value (Signaling)")] -> w674
                          frame False {
                          }
                          frame True {
                          }
                        }
                        n598 = property on="indicator_focus_status" class="Str"("Val(Sgnl)"=w674) -> ()  [unwired: 2 in, 2 out]
                      }
                    }
                  }
                }
                n599 = property on="indicator_joystick_buttons" class="Clust (strict)"("Val(Sgnl)"=w182) -> ()  [unwired: 2 in, 2 out]
                n600 = property on="indicator_joystick_axes" class="Clust (strict)"("Val(Sgnl)"=w181) -> ()  [unwired: 2 in, 2 out]
                n601 = Unbundle By Name(w171) -> ("currentXWell"=w169:i32, "currentYWell"=w167:i32, "currentXFOV"=w165:i32, "currentYFOV"=w163:i32, "currentRepeat"=w161:i32, "currentLaser"=w160:i32)
                n602 = Unbundle By Name(w172) -> ("numXWells"=w170:i32, "numYWells"=w168:i32, "numXFOVs"=w166:i32, "numYFOVs"=w164:i32, "numRepeats"=w162:i32, "numLasers"=w145:i32)
                n603 = Not Equal?(x=w119, y="Locked") -> (x != y?=w115:bool)
                n604 = And(x=w120, y=w121) -> (x .and. y?=w93:bool)
                n605 = Unbundle By Name(w110) -> ("x"=w109:i64, "y"=w108:i64, "z"=w107:i64)
                n606 = case shown="True" w91 {
                  tunnel: w101 -> [_ w697]
                  tunnel: w134 -> [_ w698]
                  frame False {
                  }
                  frame True {
                    # "Moving X Positioners When Left Thumbstick is Dragged Right or Left"
                    n607 = call "Positioner Control.vi"("control_positioner_reference"=w697, "mode"="Incremental", "index"=w698, "control_move_direction"="x", "control_request"="Write") -> ()  [unwired: 1 in, 6 out]
                  }
                }
                n608 = case shown="True" w90 {
                  tunnel: w101 -> [_ w692]
                  tunnel: w131 -> [_ w693]
                  frame False {
                  }
                  frame True {
                    # "Moving Y Positioners When Left Thumbstick is Dragged Up or Down"
                    n609 = call "Positioner Control.vi"("control_positioner_reference"=w692, "mode"="Incremental", "index"=w693, "control_move_direction"="y", "control_request"="Write") -> ()  [unwired: 1 in, 6 out]
                  }
                }
                n610 = Unbundle By Name(w150) -> ("indicator_camera_reference"=w149:refnum<k24>)
                n611 = And(x=w114, y=w115) -> (x .and. y?=w113:bool)
                n612 = And(x=w117, y=w115) -> (x .and. y?=w116:bool)
                n613 = Equal?(x=w170, y=w169) -> (x = y?=w159:bool)
                n614 = Equal?(x=w168, y=w167) -> (x = y?=w158:bool)
                n615 = Equal?(x=w166, y=w165) -> (x = y?=w157:bool)
                n616 = Equal?(x=w164, y=w163) -> (x = y?=w156:bool)
                n617 = Equal?(x=w162, y=w161) -> (x = y?=w155:bool)
                n618 = Equal?(x=w145, y=w160) -> (x = y?=w154:bool)
                n619 = Build Array(w109, w108, w107) -> (w100:i64[])
                n620 = case shown="False" w116 {
                  tunnel: w113 -> [w679 _]
                  tunnel: w101 -> [w678 w685]
                  tunnel: w130 -> [w677 _]
                  tunnel: w127 -> [_ w686]
                  frame False {
                    n621 = case shown="True" w679 {
                      tunnel: w677 -> [_ w684]
                      tunnel: w678 -> [_ w680]
                      frame False {
                      }
                      frame True {
                        # "Moving Z Positioners When Right Thumbstick is Dragged Up or Down (Coarse)"
                        n622 = call "Positioner Control.vi"("control_positioner_reference"=w680, "mode"="Incremental", "index"=w684, "control_move_direction"="z", "control_request"="Write") -> ()  [unwired: 1 in, 6 out]
                      }
                    }
                  }
                  frame True {
                    # "Moving Z Positioners When Left Thumbstick is Dragged Left or Right (Fine)"
                    n623 = Multiply(x=w686, y=0.02) -> (x*y=w687:dbl)
                    n624 = call "Positioner Control.vi"("control_positioner_reference"=w685, "mode"="Incremental", "index"=w687, "control_move_direction"="z", "control_request"="Write") -> ()  [unwired: 1 in, 6 out]
                  }
                }
                n625 = property on="indicator_positioner_current_position" class="Arr (strict)"("Val(Sgnl)"=w100) -> ()  [unwired: 2 in, 2 out]
                n626 = Build Array(w159, w158, w157, w156, w155, w154) -> (w153:bool[])
                n627 = call "Camera Control.vi"("control_request"="Is Idle", "control_camera_reference"=w149) -> ("Is Idle"=w147:bool)  [unwired: 9 in, 4 out]
                n628 = property on="indicator_message" class="Str"() -> ("Value"=w152:string)  [unwired: 2 in, 2 out]
                n629 = Equal?(x="Acquiring", y=w152) -> (x = y?=w148:bool)
                n630 = feedback #1() -> (w141:path)  [unwired: 1 in]
                n631 = Equal?(x=w143, y=w141) -> (x = y?=w144:bool)
                n632 = case shown="False" w144 {
                  tunnel: [w878 w880] -> w142
                  tunnel: w143 -> [w878 w880]
                  frame False {
                    n633 = property on="indicator_current_folder" class="DigNum (strict)"("Val(Sgnl)"=u64 0 ("Value (Signaling)")) -> ()  [unwired: 2 in, 2 out]
                  }
                  frame True {
                    # "Initializing Current Folder to 'Zero' When Saving Path Control is Changed by User"
                  }
                }
                n634 = feedback-in #1(w142) -> ()
                n635 = And Array Elements(Boolean array=w153) -> (logical AND=w146:bool)
                n636 = Build Array(w148, w146, w147) -> (w173:bool[])
                n637 = And Array Elements(Boolean array=w173) -> (logical AND=w174:bool)
                n638 = case shown="True" w174 {
                  tunnel: w148 -> [w883 _]
                  tunnel: w147 -> [w886 _]
                  tunnel: w146 -> [w890 _]
                  frame False {
                    n639 = Not(x=w886) -> (.not. x?=w882:bool)
                    n640 = Not(x=w890) -> (.not. x?=w889:bool)
                    n641 = Build Array(w883, w886, w889) -> (w888:bool[])
                    n642 = property on="control_sequence" class="Bool (strict)"() -> ("Value"=w881:bool)  [unwired: 2 in, 2 out]
                    n643 = And Array Elements(Boolean array=w888) -> (logical AND=w887:bool)
                    n644 = case shown="False" w887 {
                      frame False {
                      }
                      frame True {
                        n645 = stacked-sequence {
                          frame #0 {
                            n646 = property on="indicator_devices_reference" class="Clust (strict)"() -> ("Value"=w919:T2)  [unwired: 2 in, 2 out]
                            n647 = Unbundle By Name(w919) -> ("indicator_light_source_channel_0_reference"=w918:u64, "indicator_light_source_channel_1_reference"=w917:u64, "indicator_light_source_channel_2_reference"=w916:u64, "indicator_light_source_channel_3_reference"=w915:u64, "indicator_light_source_LED_reference"=w914:u64, "indicator_light_source_vibrator_reference"=w913:u64)
                            n648 = call "Laser Control.vi"("control_laser_source_channel_0_reference"=w918, "control_laser_source_LED_reference"=w913, "control_request"="Write", "control_laser_source_channel_1_reference"=w917, "control_laser_source_channel_2_reference"=w916, "control_laser_source_channel_3_reference"=w915, "control_laser_source_vibrator_reference"=w914, "control_laser_source"="None") -> ()  [unwired: 1 in, 7 out]
                          }
                          frame #1 {
                            n649 = property on="indicator_saved_positions" class="Arr (strict)"() -> ("Value"=w922:i64[][])  [unwired: 2 in, 2 out]
                            n650 = property on="indicator_sequence_current_parameters" class="Clust (strict)"() -> ("Value"=w935:T3)  [unwired: 2 in, 2 out]
                            n651 = property on="indicator_sequence_parameters" class="Clust (strict)"() -> ("Value"=w936:T4)  [unwired: 2 in, 2 out]
                            n652 = property on="control_sequence_file_path" class="Path"() -> ("Value"=w937:path)  [unwired: 2 in, 2 out]
                            n653 = Array Size(array=w922) -> (size(s)=w934:i32[])
                            n654 = Index Array(array=w934, index=0) -> (element=w932:i32)
                            n655 = Greater Than 0?(x=w932) -> (x > 0?=w923:bool)
                            n656 = call "Sequence Module.vi"("control_request"="Process", "control_sequence_file_path"=w937, "control_sequence_parameters"=w936, "control_sequence_current_parameters"=w935) -> ("indicator_sequence_current_parameters"=w921:T3, "indicator_sequence_move_x"=w931:bool, "indicator_sequence_move_y"=w929:bool, "indicator_sequence_distance_y"=w925:dbl, "indicator_sequence_distance_x"=w927:dbl)  [unwired: 4 in, 3 out]
                            n657 = property on="indicator_sequence_current_parameters" class="Clust (strict)"("Val(Sgnl)"=w921) -> ()  [unwired: 2 in, 2 out]
                            n658 = case shown="True" w923 {
                              tunnel: w931 -> [w942 _]
                              tunnel: [w942 w961] -> w930
                              tunnel: [w941 w961] -> w928
                              tunnel: w929 -> [w941 _]
                              tunnel: w927 -> [w940 _]
                              tunnel: [w940 w950] -> w926
                              tunnel: w925 -> [w939 _]
                              tunnel: [w939 w946] -> w924
                              tunnel: w922 -> [_ w958]
                              tunnel: w921 -> [_ w943]
                              frame False {
                              }
                              frame True {
                                w947 = 1000000.0 ("y")
                                w961 = TRUE ("indicator_sequence_move_x")
                                n659 = Unbundle By Name(w943) -> ("currentYWell"=w945:i32)
                                n660 = Decrement(x=w945) -> (x-1=w944:i32)
                                n661 = property on="indicator_positioner_current_position" class="Arr (strict)"() -> ("Value"=w956:i64[])  [unwired: 2 in, 2 out]
                                n662 = Index Array(array=w958, index (row)=w944, index (col)=0 ("disabled index (col)")) -> (element=w953:i64)
                                n663 = Index Array(array=w958, index (row)=w944, index (col)=1 ("disabled index (col)")) -> (element=w951:i64)
                                n664 = Index Array(array=w956, index=0) -> (element=w954:i64)
                                n665 = Index Array(array=w956, index=1) -> (element=w952:i64)
                                n666 = Subtract(x=w953, y=w954) -> (x-y=w949:i64)
                                n667 = Subtract(x=w951, y=w952) -> (x-y=w948:i64)
                                n668 = Divide(x=w949, y=w947) -> (x/y=w950:dbl)
                                n669 = Divide(x=w948, y=w947) -> (x/y=w946:dbl)
                              }
                            }
                            n670 = property on="indicator_sequence_distance_x" class="DigNum (strict)"("Val(Sgnl)"=w926) -> ()  [unwired: 2 in, 2 out]
                            n671 = property on="indicator_sequence_move_x" class="Bool (strict)"("Val(Sgnl)"=w930) -> ()  [unwired: 2 in, 2 out]
                            n672 = property on="indicator_sequence_distance_y" class="DigNum (strict)"("Val(Sgnl)"=w924) -> ()  [unwired: 2 in, 2 out]
                            n673 = property on="indicator_sequence_move_y" class="Bool (strict)"("Val(Sgnl)"=w928) -> ()  [unwired: 2 in, 2 out]
                          }
                          frame #2 {
                            n674 = property on="indicator_message" class="Str"("Val(Sgnl)"="Setting acquisition" ("Value (Signaling)")) -> ()  [unwired: 2 in, 2 out]
                          }
                        }
                      }
                    }
                    n675 = Build Array(w883, w882, w881) -> (w884:bool[])
                    n676 = And Array Elements(Boolean array=w884) -> (logical AND=w885:bool)
                    n677 = case shown="False" w885 {
                      frame False {
                      }
                      frame True {
                        n678 = Tick Count (ms)() -> (millisecond timer value=w894:u32)
                        n679 = Divide(x=w894, y=u32 1000) -> (x/y=w896:dbl)
                        n680 = property on="indicator_acquisition_start_time" class="DigNum (strict)"() -> ("Value"=w891:dbl)  [unwired: 2 in, 2 out]
                        n681 = property on="indicator_UV_activation_time" class="DigNum (strict)"() -> ("Value"=w897:dbl)  [unwired: 2 in, 2 out]
                        n682 = Subtract(x=w896, y=w891) -> (x-y=w901:dbl)
                        n683 = Round To Nearest(number=w901) -> (nearest integer value=w902:dbl)
                        n684 = Multiply(x=w897, y=60.0) -> (x*y=w899:dbl)
                        n685 = Quotient & Remainder(x=w902, y=w899) -> (x-y*floor(x/y)=w892:dbl, floor(x/y)=w900:dbl)
                        n686 = Equal To 0?(x=w892) -> (x = 0?=w893:bool)
                        n687 = case shown="True" w893 {
                          tunnel: w900 -> [_ w911]
                          frame False {
                          }
                          frame True {
                            n688 = property on="indicator_UV_activation_intensity" class="DigNum (strict)"() -> ("Value"=w910:dbl)  [unwired: 2 in, 2 out]
                            n689 = property on="indicator_devices_reference" class="Clust (strict)"() -> ("Value"=w909:T11)  [unwired: 2 in, 2 out]
                            n690 = Multiply(x=w911, y=w910) -> (x*y=w904:dbl)
                            n691 = Unbundle By Name(w909) -> ("indicator_light_source_channel_0_reference"=w907:u64)
                            n692 = In Range and Coerce(upper limit=5.0, x=w904, lower limit=0.0) -> (coerced(x)=w903:dbl)  [unwired: 1 out]
                            n693 = call "Laser Control.vi"("control_laser_source_channel_0_reference"=w907, "control_request"="Activate", "control_laser_source_power"=w903) -> ()  [unwired: 6 in, 7 out]
                          }
                        }
                      }
                    }
                  }
                  frame True {
                    # "Terminating Acquisition"
                    n694 = stacked-sequence {
                      frame #0 {
                        n695 = property on="indicator_devices_reference" class="Clust (strict)"() -> ("Value"=w970:T2)  [unwired: 2 in, 2 out]
                        n696 = Unbundle By Name(w970) -> ("indicator_light_source_channel_0_reference"=w969:u64, "indicator_light_source_channel_1_reference"=w968:u64, "indicator_light_source_channel_2_reference"=w967:u64, "indicator_light_source_channel_3_reference"=w966:u64, "indicator_light_source_LED_reference"=w965:u64, "indicator_light_source_vibrator_reference"=w964:u64)
                        n697 = call "Laser Control.vi"("control_laser_source_channel_0_reference"=w969, "control_laser_source_LED_reference"=w964, "control_request"="Write", "control_laser_source_channel_1_reference"=w968, "control_laser_source_channel_2_reference"=w967, "control_laser_source_channel_3_reference"=w966, "control_laser_source_vibrator_reference"=w965, "control_laser_source"="None") -> ()  [unwired: 1 in, 7 out]
                      }
                      frame #1 {
                        n698 = property on="indicator_message" class="Str"("Val(Sgnl)"="Ready" ("Value (Signaling)")) -> ()  [unwired: 2 in, 2 out]
                      }
                    }
                  }
                }
                n699 = feedback #2() -> (w88:i16)  [unwired: 1 in]
                n700 = case shown="True" w93 {
                  tunnel: w92 -> [w440 w450]
                  tunnel: [w440 w451] -> w87
                  tunnel: w88 -> [_ w451]
                  tunnel: w89 -> [_ _]
                  tunnel: w91 -> [_ w444]
                  tunnel: w90 -> [_ w443]
                  tunnel: [i16 0 w441] -> _
                  frame False {
                  }
                  frame True {
                    # "Autofocusing loop"
                    n701 = Or(x=w444, y=w443) -> (x .or. y?=w445:bool)
                    n702 = Subtract(x=w451, y=w450) -> (x-y=w441:i16)
                    n703 = property on="indicator_error" class="DigNum (strict)"("Val(Sgnl)"=w441) -> ()  [unwired: 2 in, 2 out]
                    n704 = case shown="False" w445 {
                      tunnel: [i16 30 ("y") i16 150 ("y")] -> w442
                      frame False {
                      }
                      frame True {
                      }
                    }
                    n705 = To Quad Integer(1:w441) -> (0:w447:i64)
                    n706 = property on="indicator_devices_reference" class="Clust (strict)"() -> ("Value"=w453:T11)  [unwired: 2 in, 2 out]
                    n707 = To Quad Integer(1:w442) -> (0:w446:i64)
                    n708 = Multiply(x=w447, y=w446) -> (x*y=w449:i64)
                    n709 = Unbundle By Name(w453) -> ("indicator_positioner_reference"=w452:refnum<class "SA_CTL.lvclass">)
                    n710 = To Quad Integer(1:w449) -> (0:w448:i64)
                    n711 = call "Positioner Control.vi"("control_move_length"=w448, "control_positioner_reference"=w452, "mode"="Set", "control_move_direction"="z", "control_request"="Write") -> ()  [unwired: 1 in, 6 out]
                  }
                }
                n712 = feedback-in #2(w87) -> ()
                n713 = node-c288() -> ()  [unwired: 1 in, 1 out]
              }
              n714 = node-c288(w80) -> ()  [unwired: 1 out]
            }
          }
        }
      }
    }
    frame #3 {
      w1088 = "Close" ("control_request")
      # "Closing devices"
      n715 = property on="indicator_devices_reference" class="Clust (strict)"() -> ("Value"=w1080:T11)  [unwired: 2 in, 2 out]
      n716 = Unbundle By Name(w1080) -> ("indicator_light_source_channel_0_reference"=w1086:u64, "indicator_light_source_channel_1_reference"=w1085:u64, "indicator_light_source_channel_2_reference"=w1084:u64, "indicator_light_source_channel_3_reference"=w1083:u64, "indicator_light_source_LED_reference"=w1076:u64, "indicator_light_source_LED_reference 2"=w1075:u64, "indicator_library_reference"=w1081:refnum<k24>, "indicator_camera_reference"=w1087:refnum<k24>, "indicator_positioner_reference"=w1082:refnum<class "SA_CTL.lvclass">)  [unwired: 1 out]
      n717 = call "Joystick Control.vi"("control_request"=w1088, "control_devices_reference"=w1080) -> ()  [unwired: 5 in, 5 out]
      n718 = call "Filter Control.vi"("control_request"=w1088) -> ()  [unwired: 10 in, 1 out]
      n719 = call "Detector Control.vi"("control_request"=w1088) -> ()  [unwired: 9 in, 2 out]
      n720 = property on="indicator_main_light sources_status" class="Bool (strict)"() -> ("Value"=w1078:bool)  [unwired: 2 in, 2 out]
      n721 = property on="indicator_main_positioner_status" class="Bool (strict)"() -> ("Value"=w1079:bool)  [unwired: 2 in, 2 out]
      n722 = property on="indicator_main_camera_status" class="Bool (strict)"() -> ("Value"=w1077:bool)  [unwired: 2 in, 2 out]
      n723 = flat-sequence {
        tunnel: w1088 -> [w1100]
        tunnel: w1087 -> [w1099]
        tunnel: w1077 -> [w1098]
        tunnel: w1081 -> [w1103]
        frame #0 {
          n724 = case shown="True" w1098 {
            tunnel: w1100 -> [_ w1102]
            tunnel: w1099 -> [_ w1101]
            frame False {
            }
            frame True {
              n725 = call "Camera Control.vi"("control_request"=w1102, "control_camera_reference"=w1101) -> ()  [unwired: 9 in, 5 out]
            }
          }
        }
        frame #1 {
          n726 = call "Camera Control.vi"("control_request"="Release", "control_library_reference"=w1103) -> ()  [unwired: 9 in, 5 out]
        }
      }
      n727 = case shown="True" w1079 {
        tunnel: w1088 -> [_ w1097]
        tunnel: w1082 -> [_ w1096]
        frame False {
        }
        frame True {
          n728 = call "Positioner Control.vi"("control_positioner_reference"=w1096, "control_request"=w1097) -> ()  [unwired: 4 in, 6 out]
        }
      }
      n729 = case shown="True" w1078 {
        tunnel: w1088 -> [_ w1095]
        tunnel: w1086 -> [_ w1094]
        tunnel: w1085 -> [_ w1093]
        tunnel: w1084 -> [_ w1092]
        tunnel: w1083 -> [_ w1091]
        tunnel: w1076 -> [_ w1090]
        tunnel: w1075 -> [_ w1089]
        frame False {
        }
        frame True {
          n730 = call "Laser Control.vi"("control_laser_source_channel_0_reference"=w1094, "control_laser_source_LED_reference"=w1089, "control_request"=w1095, "control_laser_source_channel_1_reference"=w1093, "control_laser_source_channel_2_reference"=w1092, "control_laser_source_channel_3_reference"=w1091, "control_laser_source_vibrator_reference"=w1090) -> ()  [unwired: 2 in, 7 out]
        }
      }
    }
  }
